vi "main.vi"() -> ()   [LabVIEW 2020]
uses:
  <vilib>/Platform/TimedLoop/XDataNode/timing_clust.ctl
  <vilib>/Platform/TimedLoop/XDataNode/nitl_modes.ctl
  <vilib>/Platform/TimedLoop/XDataNode/wakeup.ctl
  <vilib>/addons/control/pid/pid.llb/PID (DBL).vi
  <vilib>/imath/engines/lvmath2/RunTimeEngine/IndexReplace/NIMS M($,S)=V.vi
  <instcachedir>/0/NIMS M($,S)=V_85A28EB895514E96A13A10261726EE3A.lvgen/NIMS M($,S)=V_85A28EB895514E96A13A10261726EE3A_001.vi
  <vilib>/imathl/engines/lvmath/Functions/Error Handling/Create Error.vi
  <vilib>/imath/engines/lvmath2/RunTimeEngine/BuiltInFunctions/diag/NIMS_diag.vi
  <instcachedir>/0/NIMS_diag_5DC8FB40F025456A81838E2C880FD792.lvgen/NIMS_diag_5DC8FB40F025456A81838E2C880FD792_003.vi
  <vilib>/imath/engines/lvmath2/RunTimeEngine/NodeEndStatement/NIMS_NodeEndStatement_Output.vi
  <instcachedir>/0/NIMS_NodeEndStatement_Output_53EC0D466D134D7ABD903AC30B43404B.lvgen/NIMS_NodeEndStatement_Output_53EC0D466D134D7ABD903AC30B43404B_005.vi
  <instcachedir>/0/NIMS_NodeEndStatement_Output_53EC0D466D134D7ABD903AC30B43404B.lvgen/NIMS_NodeEndStatement_Output_53EC0D466D134D7ABD903AC30B43404B_010.vi
  <vilib>/imath/engines/lvmath2/RunTimeEngine/ErrorHandling/NIMS_Finalize Error.vi
  <vilib>/imath/engines/lvmath2/RunTimeEngine/IndexRead/NIMS V(S).vi
  <instcachedir>/0/NIMS V(S)_0488751826AF41519A22953C041130DC.lvgen/NIMS V(S)_0488751826AF41519A22953C041130DC_000.vi
  <vilib>/imath/engines/lvmath2/RunTimeEngine/ErrorHandling/NIMS_Create Error From Enums.vi
  <vilib>/imath/engines/lvmath2/RunTimeEngine/RangeToken/NIMS_Range_R2 - Integer.vi
  <instcachedir>/0/NIMS_Range_R2 - Integer_FFC1A4B1B9F04947ABCB56F009996D55.lvgen/NIMS_Range_R2 - Integer_FFC1A4B1B9F04947ABCB56F009996D55_000.vi
  <vilib>/imath/engines/lvmath2/RunTimeEngine/CommandStatement/MC_CommandStatement_break.vi
  <vilib>/imath/engines/lvmath2/RunTimeEngine/VariableToken/NIMS_VariableToken_CondDefinedDefinedByReplace.vi
  <instcachedir>/0/NIMS_VariableToken_CondDefinedDefinedByReplace_D162CFFC24174562A9FEA619A91E1A56.lvgen/NIMS_VariableToken_CondDefinedDefinedByReplace_D162CFFC24174562A9FEA619A91E1A56_000.vi
  <vilib>/imath/engines/lvmath2/RunTimeEngine/IndexReplace/NIMS V(S)=S.vi
  <instcachedir>/0/NIMS V(S)=S_36728E0438CF49488BD4AB9ABCA5ECA4.lvgen/NIMS V(S)=S_36728E0438CF49488BD4AB9ABCA5ECA4_001.vi
  <vilib>/imath/engines/lvmath2/RunTimeEngine/VariableToken/NIMS_VariableToken_CondDefined.vi
  <instcachedir>/0/NIMS_VariableToken_CondDefined_537E119D71C74F9D9452D6FF923F1E1F.lvgen/NIMS_VariableToken_CondDefined_537E119D71C74F9D9452D6FF923F1E1F_000.vi
  <vilib>/imath/engines/lvmath2/RunTimeEngine/IndexRead/NIMS V($).vi
  <instcachedir>/0/NIMS V($)_C593F32C7F6B43C7B1793952E292524F.lvgen/NIMS V($)_C593F32C7F6B43C7B1793952E292524F_000.vi
  <vilib>/imath/engines/lvmath2/RunTimeEngine/ArithmeticOperatorToken/NIMS_ArithmeticOperator_rightdiv(C,C).vi
  <instcachedir>/0/NIMS_ArithmeticOperator_rightdiv(C,C)_34A6183377BA4447889BB2F60308B12E.lvgen/NIMS_ArithmeticOperator_rightdiv(C,C)_34A6183377BA4447889BB2F60308B12E_000.vi
  <instcachedir>/0/NIMS_diag_5DC8FB40F025456A81838E2C880FD792.lvgen/NIMS_diag_5DC8FB40F025456A81838E2C880FD792_002.vi
  <vilib>/imath/engines/lvmath2/RunTimeEngine/ArithmeticOperatorToken/NIMS_ArithmeticOperator_minus.vi
  <instcachedir>/0/NIMS_ArithmeticOperator_minus_822089A08BE049DB927E6BEA78E100F1.lvgen/NIMS_ArithmeticOperator_minus_822089A08BE049DB927E6BEA78E100F1_009.vi
  <vilib>/imath/engines/lvmath2/RunTimeEngine/ArithmeticOperatorToken/NIMS_ArithmeticOperator_times.vi
  <instcachedir>/0/NIMS_ArithmeticOperator_times_E1747072C05B43E9AAEA71FEEAEB18C8.lvgen/NIMS_ArithmeticOperator_times_E1747072C05B43E9AAEA71FEEAEB18C8_002.vi
  <vilib>/imath/engines/lvmath2/RunTimeEngine/ArithmeticOperatorToken/NIMS_ArithmeticOperator_plus.vi
  <instcachedir>/0/NIMS_ArithmeticOperator_plus_54468E2FAC2848C4BF0D457641184E60.lvgen/NIMS_ArithmeticOperator_plus_54468E2FAC2848C4BF0D457641184E60_005.vi
  <instcachedir>/0/NIMS_ArithmeticOperator_minus_822089A08BE049DB927E6BEA78E100F1.lvgen/NIMS_ArithmeticOperator_minus_822089A08BE049DB927E6BEA78E100F1_004.vi
  <instcachedir>/0/NIMS_ArithmeticOperator_plus_54468E2FAC2848C4BF0D457641184E60.lvgen/NIMS_ArithmeticOperator_plus_54468E2FAC2848C4BF0D457641184E60_001.vi
  <instcachedir>/0/NIMS V($)_C593F32C7F6B43C7B1793952E292524F.lvgen/NIMS V($)_C593F32C7F6B43C7B1793952E292524F_001.vi
  <instcachedir>/0/NIMS_ArithmeticOperator_minus_822089A08BE049DB927E6BEA78E100F1.lvgen/NIMS_ArithmeticOperator_minus_822089A08BE049DB927E6BEA78E100F1_003.vi
  <instcachedir>/0/NIMS_ArithmeticOperator_plus_54468E2FAC2848C4BF0D457641184E60.lvgen/NIMS_ArithmeticOperator_plus_54468E2FAC2848C4BF0D457641184E60_004.vi
  <instcachedir>/0/NIMS V(S)=S_36728E0438CF49488BD4AB9ABCA5ECA4.lvgen/NIMS V(S)=S_36728E0438CF49488BD4AB9ABCA5ECA4_000.vi
  <instcachedir>/0/NIMS_ArithmeticOperator_times_E1747072C05B43E9AAEA71FEEAEB18C8.lvgen/NIMS_ArithmeticOperator_times_E1747072C05B43E9AAEA71FEEAEB18C8_000.vi
  <vilib>/imath/engines/lvmath2/RunTimeEngine/ArithmeticOperatorToken/NIMS_ArithmeticOperator_multmx(M,CV).vi
  <instcachedir>/0/NIMS_ArithmeticOperator_multmx(M,CV)_6A1ED936907E4DE39F29C31CF1EB9098.lvgen/NIMS_ArithmeticOperator_multmx(M,CV)_6A1ED936907E4DE39F29C31CF1EB9098_000.vi
  <vilib>/imath/engines/lvmath2/RunTimeEngine/ArithmeticOperatorToken/NIMS_ArithmeticOperator_multmx(M,CV)-internal.vi
  <instcachedir>/0/NIMS_ArithmeticOperator_multmx(M,CV)-internal_19A14CC5BE0A4D31BE1E94A2E998D8C3.lvgen/NIMS_ArithmeticOperator_multmx(M,CV)-internal_19A14CC5BE0A4D31BE1E94A2E998D8C3_001.vi
  <instcachedir>/0/NIMS_ArithmeticOperator_plus_54468E2FAC2848C4BF0D457641184E60.lvgen/NIMS_ArithmeticOperator_plus_54468E2FAC2848C4BF0D457641184E60_003.vi
  <instcachedir>/0/NIMS_ArithmeticOperator_plus_54468E2FAC2848C4BF0D457641184E60.lvgen/NIMS_ArithmeticOperator_plus_54468E2FAC2848C4BF0D457641184E60_010.vi
  <instcachedir>/0/NIMS_ArithmeticOperator_minus_822089A08BE049DB927E6BEA78E100F1.lvgen/NIMS_ArithmeticOperator_minus_822089A08BE049DB927E6BEA78E100F1_010.vi
  <vilib>/imath/engines/lvmath2/RunTimeEngine/ArithmeticOperatorToken/NIMS_ArithmeticOperator_multmx.vi
  <instcachedir>/0/NIMS_ArithmeticOperator_multmx_177F0753FB7A49B190E35F5DD0E80316.lvgen/NIMS_ArithmeticOperator_multmx_177F0753FB7A49B190E35F5DD0E80316_003.vi
  <instcachedir>/0/NIMS_ArithmeticOperator_multmx(M,CV)_6A1ED936907E4DE39F29C31CF1EB9098.lvgen/NIMS_ArithmeticOperator_multmx(M,CV)_6A1ED936907E4DE39F29C31CF1EB9098_003.vi
  <instcachedir>/0/NIMS_ArithmeticOperator_times_E1747072C05B43E9AAEA71FEEAEB18C8.lvgen/NIMS_ArithmeticOperator_times_E1747072C05B43E9AAEA71FEEAEB18C8_011.vi
  <instcachedir>/0/NIMS_ArithmeticOperator_plus_54468E2FAC2848C4BF0D457641184E60.lvgen/NIMS_ArithmeticOperator_plus_54468E2FAC2848C4BF0D457641184E60_002.vi
  <instcachedir>/0/NIMS_ArithmeticOperator_minus_822089A08BE049DB927E6BEA78E100F1.lvgen/NIMS_ArithmeticOperator_minus_822089A08BE049DB927E6BEA78E100F1_011.vi
  <vilib>/imath/engines/lvmath2/RunTimeEngine/ArithmeticOperatorToken/NIMS_ArithmeticOperator_rightdiv.vi
  <instcachedir>/0/NIMS_ArithmeticOperator_rightdiv_8260AC44E1124B869C886786403FE7FC.lvgen/NIMS_ArithmeticOperator_rightdiv_8260AC44E1124B869C886786403FE7FC_000.vi
  <instcachedir>/0/NIMS_ArithmeticOperator_multmx(M,CV)_6A1ED936907E4DE39F29C31CF1EB9098.lvgen/NIMS_ArithmeticOperator_multmx(M,CV)_6A1ED936907E4DE39F29C31CF1EB9098_001.vi
  <instcachedir>/0/NIMS_ArithmeticOperator_plus_54468E2FAC2848C4BF0D457641184E60.lvgen/NIMS_ArithmeticOperator_plus_54468E2FAC2848C4BF0D457641184E60_011.vi
  <instcachedir>/0/NIMS_ArithmeticOperator_minus_822089A08BE049DB927E6BEA78E100F1.lvgen/NIMS_ArithmeticOperator_minus_822089A08BE049DB927E6BEA78E100F1_008.vi
  <instcachedir>/0/NIMS_ArithmeticOperator_times_E1747072C05B43E9AAEA71FEEAEB18C8.lvgen/NIMS_ArithmeticOperator_times_E1747072C05B43E9AAEA71FEEAEB18C8_012.vi
  <instcachedir>/0/NIMS_ArithmeticOperator_rightdiv(C,C)_34A6183377BA4447889BB2F60308B12E.lvgen/NIMS_ArithmeticOperator_rightdiv(C,C)_34A6183377BA4447889BB2F60308B12E_001.vi
  <vilib>/imath/engines/lvmath2/RunTimeEngine/MatrixToken/NIMS_MatrixToken_SorCV_M.vi
  <instcachedir>/0/NIMS_MatrixToken_SorCV_M_84289C48EDA3463080C22A503926496B.lvgen/NIMS_MatrixToken_SorCV_M_84289C48EDA3463080C22A503926496B_000.vi
  <instcachedir>/0/NIMS_ArithmeticOperator_minus_822089A08BE049DB927E6BEA78E100F1.lvgen/NIMS_ArithmeticOperator_minus_822089A08BE049DB927E6BEA78E100F1_002.vi
  <instcachedir>/0/NIMS_MatrixToken_SorCV_M_84289C48EDA3463080C22A503926496B.lvgen/NIMS_MatrixToken_SorCV_M_84289C48EDA3463080C22A503926496B_001.vi
  <instcachedir>/0/NIMS_ArithmeticOperator_plus_54468E2FAC2848C4BF0D457641184E60.lvgen/NIMS_ArithmeticOperator_plus_54468E2FAC2848C4BF0D457641184E60_000.vi
  <vilib>/imath/engines/lvmath2/RunTimeEngine/IndexRead/NIMS V(R2).vi
  <instcachedir>/0/NIMS V(R2)_C76619605A0E4E9F8B2FA9389712AC47.lvgen/NIMS V(R2)_C76619605A0E4E9F8B2FA9389712AC47_000.vi
  <instcachedir>/0/NIMS V(R2)_C76619605A0E4E9F8B2FA9389712AC47.lvgen/NIMS V(R2)_C76619605A0E4E9F8B2FA9389712AC47_001.vi
  <vilib>/imath/engines/lvmath2/RunTimeEngine/BuiltInFunctions/reshapemx/NIMS_[GM]_reshapemx.vi
  <instcachedir>/0/NIMS_[GM]_reshapemx_98F4FEDA5D2741A4824CEDFB6097FB68.lvgen/NIMS_[GM]_reshapemx_98F4FEDA5D2741A4824CEDFB6097FB68_004.vi
  <vilib>/imath/engines/lvmath2/RunTimeEngine/IndexRead/NIMS M(S,$).vi
  <instcachedir>/0/NIMS M(S,$)_F24F360562DE41D8BE234322A2E15C65.lvgen/NIMS M(S,$)_F24F360562DE41D8BE234322A2E15C65_001.vi
  <vilib>/imath/engines/lvmath2/RunTimeEngine/ArithmeticOperatorToken/NIMS_ArithmeticOperator_multmx(RV,CV).vi
  <instcachedir>/0/NIMS_ArithmeticOperator_multmx(RV,CV)_B88EFA1B0B8541B182B3EADCEACED710.lvgen/NIMS_ArithmeticOperator_multmx(RV,CV)_B88EFA1B0B8541B182B3EADCEACED710_001.vi
  <instcachedir>/0/NIMS V(S)_0488751826AF41519A22953C041130DC.lvgen/NIMS V(S)_0488751826AF41519A22953C041130DC_003.vi
  <vilib>/imath/engines/lvmath2/RunTimeEngine/IndexReplace/NIMS V(S)=M.vi
  <instcachedir>/0/NIMS V(S)=M_4F924C5350174586BCA8F9B45EA0F965.lvgen/NIMS V(S)=M_4F924C5350174586BCA8F9B45EA0F965_001.vi
  <vilib>/imath/engines/lvmath2/RunTimeEngine/IndexRead/NIMS M(S).vi
  <instcachedir>/0/NIMS M(S)_B826C018497E4940AE96BD27B540B6FB.lvgen/NIMS M(S)_B826C018497E4940AE96BD27B540B6FB_004.vi
  <instcachedir>/0/NIMS_ArithmeticOperator_multmx(RV,CV)_B88EFA1B0B8541B182B3EADCEACED710.lvgen/NIMS_ArithmeticOperator_multmx(RV,CV)_B88EFA1B0B8541B182B3EADCEACED710_000.vi
  <vilib>/imath/engines/lvmath2/RunTimeEngine/ArithmeticOperatorToken/NIMS_ArithmeticOperator_rightdivmx(C,C).vi
  <instcachedir>/0/NIMS_ArithmeticOperator_rightdivmx(C,C)_00A7E666A69647418148ACDCFFBCE354.lvgen/NIMS_ArithmeticOperator_rightdivmx(C,C)_00A7E666A69647418148ACDCFFBCE354_000.vi
  <vilib>/imath/engines/lvmath2/RunTimeEngine/ArithmeticOperatorToken/NIMS_ArithmeticOperator_multmx(RV,CV)-internal.vi
  <instcachedir>/0/NIMS_ArithmeticOperator_multmx(RV,CV)-internal_E772CF64F86B43F3BAB2B4FC2EB32E29.lvgen/NIMS_ArithmeticOperator_multmx(RV,CV)-internal_E772CF64F86B43F3BAB2B4FC2EB32E29_002.vi
  <vilib>/imath/engines/lvmath2/RunTimeEngine/BuiltInFunctions/max/2 inputs/NIMS_max(CG,CG)-no size check.vi
  <instcachedir>/0/NIMS_max(CG,CG)-no size check_4775AE88A51C4793B48F105C5674D795.lvgen/NIMS_max(CG,CG)-no size check_4775AE88A51C4793B48F105C5674D795_000.vi
  <vilib>/imath/engines/lvmath2/RunTimeEngine/BuiltInFunctions/min/2 inputs/NIMS_min(CG,CG)-no size check.vi
  <instcachedir>/0/NIMS_min(CG,CG)-no size check_E9FF1D1EB4794D67BF6952418B074C1B.lvgen/NIMS_min(CG,CG)-no size check_E9FF1D1EB4794D67BF6952418B074C1B_000.vi
  <instcachedir>/0/NIMS V(S)_0488751826AF41519A22953C041130DC.lvgen/NIMS V(S)_0488751826AF41519A22953C041130DC_002.vi
  <instcachedir>/0/NIMS_max(CG,CG)-no size check_4775AE88A51C4793B48F105C5674D795.lvgen/NIMS_max(CG,CG)-no size check_4775AE88A51C4793B48F105C5674D795_001.vi
  <instcachedir>/0/NIMS_min(CG,CG)-no size check_E9FF1D1EB4794D67BF6952418B074C1B.lvgen/NIMS_min(CG,CG)-no size check_E9FF1D1EB4794D67BF6952418B074C1B_001.vi
  <instcachedir>/0/NIMS_diag_5DC8FB40F025456A81838E2C880FD792.lvgen/NIMS_diag_5DC8FB40F025456A81838E2C880FD792_004.vi
  <instcachedir>/0/NIMS_ArithmeticOperator_multmx_177F0753FB7A49B190E35F5DD0E80316.lvgen/NIMS_ArithmeticOperator_multmx_177F0753FB7A49B190E35F5DD0E80316_006.vi
  <instcachedir>/0/NIMS M(S)_B826C018497E4940AE96BD27B540B6FB.lvgen/NIMS M(S)_B826C018497E4940AE96BD27B540B6FB_000.vi
  <vilib>/imath/engines/lvmath2/RunTimeEngine/IndexReplace/NIMS M(S)=S.vi
  <instcachedir>/0/NIMS M(S)=S_033E230F5F1E47BAA81748F03F1A64B6.lvgen/NIMS M(S)=S_033E230F5F1E47BAA81748F03F1A64B6_001.vi
  <instcachedir>/0/NIMS M(S)=S_033E230F5F1E47BAA81748F03F1A64B6.lvgen/NIMS M(S)=S_033E230F5F1E47BAA81748F03F1A64B6_002.vi
  <instcachedir>/0/NIMS_ArithmeticOperator_times_E1747072C05B43E9AAEA71FEEAEB18C8.lvgen/NIMS_ArithmeticOperator_times_E1747072C05B43E9AAEA71FEEAEB18C8_003.vi
  <vilib>/imath/engines/lvmath2/RunTimeEngine/NodeEndStatement/NIMS_NodeEndStatement_Get Vector.vi
  <instcachedir>/0/NIMS_NodeEndStatement_Get Vector_F9EEA26507564AFBA1E30D500A99934B.lvgen/NIMS_NodeEndStatement_Get Vector_F9EEA26507564AFBA1E30D500A99934B_003.vi
  <instcachedir>/0/NIMS_NodeEndStatement_Get Vector_F9EEA26507564AFBA1E30D500A99934B.lvgen/NIMS_NodeEndStatement_Get Vector_F9EEA26507564AFBA1E30D500A99934B_001.vi
  <vilib>/imath/engines/lvmath2/RunTimeEngine/NodeEndStatement/NIMS_NodeEndStatement_Get Scalar.vi
  <instcachedir>/0/NIMS_NodeEndStatement_Get Scalar_52867EB063654D1B93D9FE1895BC48DF.lvgen/NIMS_NodeEndStatement_Get Scalar_52867EB063654D1B93D9FE1895BC48DF_000.vi
  <vilib>/imath/engines/lvmath/Functions/Error Handling/MergeErrorsWrapper.vi
  <instcachedir>/0/NIMS_NodeEndStatement_Output_53EC0D466D134D7ABD903AC30B43404B.lvgen/NIMS_NodeEndStatement_Output_53EC0D466D134D7ABD903AC30B43404B_000.vi
  <instcachedir>/0/NIMS_NodeEndStatement_Output_53EC0D466D134D7ABD903AC30B43404B.lvgen/NIMS_NodeEndStatement_Output_53EC0D466D134D7ABD903AC30B43404B_001.vi
  <instcachedir>/0/NIMS_NodeEndStatement_Output_53EC0D466D134D7ABD903AC30B43404B.lvgen/NIMS_NodeEndStatement_Output_53EC0D466D134D7ABD903AC30B43404B_009.vi
  <vilib>/Platform/TimedLoop/XDataNode/XDataNode.xnode
  <vilib>/Platform/TimedLoop/XDataNode/XDNodeRunTimeDep.lvlib
  <vilib>/addons/control/pid/NI_PID_pid.lvlib
panel:
  out "Gamma_L":dbl(graph)
  out "Load":dbl(graph)
  out "No error 3":bool
  out "No error 2":bool
  in  "Use\nPreset_Theta":bool=TRUE
  out "Theta_Boom_F_hat_next":T1(graph)
  out "Theta_Boom_Q_hat_next":T1(graph)
  out "Theta_Stick_Q_hat_next":T1(graph)
  out "Theta_Stick_F_hat_next":T1(graph)
  out "e2_e3":dbl[](array[numeric])
  out "e3":dbl[](array[numeric])
  out "e2":dbl[](array[numeric])
  out "F_Boom":cluster{dbl, dbl, dbl, dbl}(graph)
  out "Q_Swing":cluster{dbl, dbl, dbl, dbl}(graph)
  in  "保存路径":path=path "C:/Qmz/data1.bin"
  in  "Save Data":bool=TRUE
  in  "Stop\nTheta_Update":bool
  out "Q_Boom":cluster{dbl, dbl, dbl, dbl}(graph)
  out "F_Stick":cluster{dbl, dbl, dbl, dbl}(graph)
  out "Q_Stick":cluster{dbl, dbl, dbl, dbl}(graph)
  out "F_Swing":cluster{dbl, dbl, dbl, dbl}(graph)
  out "Esti_e2":T2(graph)={"FLda1[0]"=125.504748463915, "FLda1[1]"=53.955555282260676, "FLda1[2]"=-93.06627669799211}
  out "Esti_e1":T2(graph)={"FLda1[0]"=125.504748463915, "FLda1[1]"=53.955555282260676, "FLda1[2]"=-93.06627669799211}
  out "Swing":T3(graph)
  out "Stick":T3(graph)
  out "Boom":T3(graph)
  in  "sw_Y_Q":bool
  in  "w2":dbl[](array[numeric])=[1414.0, 4000.0, 3020.0]
  in  "w1":dbl[](array[numeric])=[0.26, 1.1, 0.07]
  out "Theta_Boom_Q_hat_next":dbl[](array[numeric])
  out "Theta_Boom_F_hat_next":dbl[](array[numeric])
  out "Theta_Swing_Q_hat_next":dbl[](array[numeric])
  out "Theta_Swing_F_hat_next":dbl[](array[numeric])
  out "Theta_Stick_Q_hat_next":dbl[](array[numeric])
  out "Theta_Stick_F_hat_next":dbl[](array[numeric])
  out "ARC_U":dbl[](array[numeric])
  in  "sw_d2hat":bool
  in  "sw_d1hat":bool
  in  "gamma_d2(E-8)":dbl[](array[numeric])=[6.5, 1.2, 3.5]
  in  "gamma_d1":dbl[](array[numeric])=[250.0, 6002.000000000004, 6000.1]
  in  "Theta_s2_init(E-8)":dbl[](array[numeric])=[2.0, 2.3, 2.5, 0.0, 100.0, 10.0, 0.0, -99.0, -200.0]
  in  "Theta_s1_init":dbl[](array[numeric])=[500.0, 66.0, 30.0, 53.0, 57.0, 31.0, -10.0, -73.0, 77.0]
  in  "sw_FLda1":bool=TRUE
  in  "sw_QLda1":bool=TRUE
  in  "STOP/Return to save position":bool=TRUE
  in  "Swing？(F)":bool=TRUE
  in  "Boom？(F)":bool
  in  "Stickj？(F)":bool=TRUE
  in  "K3(E-8)":dbl[](array[numeric])=[0.8, 1.0, 1.5] format="%#_8g"
  in  "K2":dbl[](array[numeric])=[650.0, 850.0, 790.0]
  in  "K1":dbl[](array[numeric])=[80.0, 80.0, 80.0]
  out "?":string="Now OpenLoop is running"
  out "?":string="Now OpenLoop is running"
  out "?":string="Now OpenLoop is running"
  in  "CloseLoop":T4 caption="ARC开关"
  out "Angle_Stick":dbl
  out "Angle_Boom":dbl
  out "Angle_Swing":dbl
  out "millisecond timer value":u32
  out "real time(s)":dbl
  out "minus":dbl format="%#_10g"
  out "No error":bool
  in  "PID gains":T5={"proportional gain (Kc)"=0.15, "integral time (Ti, min)"=0.003, "derivative time (Td, min)"=0.0005} caption="未越界" {"derivative time (Td, min)" format="%.6f"; "integral time (Ti, min)" format="%.6f"; "proportional gain (Kc)" step=0.01 format="%.6f"}
  out "?":bool
  in  "PID gains 2":T5={"proportional gain (Kc)"=0.16, "integral time (Ti, min)"=0.006, "derivative time (Td, min)"=0.0001} caption="未越界" {"derivative time (Td, min)" format="%.6f"; "integral time (Ti, min)" format="%.6f"; "proportional gain (Kc)" format="%.6f"}
  in  "PID gains 3":T5={"proportional gain (Kc)"=0.15, "integral time (Ti, min)"=0.003, "derivative time (Td, min)"=1e-05} caption="未越界" {"derivative time (Td, min)" step=0.001 format="%.6f"; "integral time (Ti, min)" step=0.001 format="%.6f"; "proportional gain (Kc)" step=0.01 format="%.6f"}
  out "?":bool
  out "?":bool
  in  "OpenLoop":T6={"Swing"=TRUE, "Boom"=TRUE, "Stick"=TRUE, "Swing_U"=-1.0, "Boom_U"=1.0, "Stick_U"=-1.0}
  in  "t-whole_Swing":i32=200
  in  "p_end Swing":dbl=-40.0
  in  "a_max Swing":dbl=-20.0
  in  "v_max Swing":dbl=-20.0
  in  "t-whole_Boom":i32=200
  in  "p_end Boom":dbl=-40.0
  in  "a_max Boom":dbl=-20.0
  in  "v_max Boom":dbl=-20.0
  in  "t-whole_Stick":i32=200
  in  "p_end_Stick":dbl=-20.0
  in  "a_max_Stick":dbl=-20.0
  in  "v_max_Stick":dbl=-20.0
  in  "pin1":dbl(slide)=-15.718390804597696 scale=-60.0..55.0
  in  "Stick":T7={"Open P2P Traj"=TRUE, "Open Sine Traj"=FALSE, "Open Ramp Traj"=FALSE, "Open DIY Traj"=FALSE}
  in  "Boom":T7={"Open P2P Traj"=TRUE, "Open Sine Traj"=FALSE, "Open Ramp Traj"=FALSE, "Open DIY Traj"=FALSE}
  in  "Swing":T7={"Open P2P Traj"=TRUE, "Open Sine Traj"=FALSE, "Open Ramp Traj"=FALSE, "Open DIY Traj"=FALSE}
  in  "pin2":dbl(slide)=69.49152542372882 scale=-20.0..90.0
  in  "pin3":dbl(slide)=-69.65868263473052 scale=-160.0..-53.0
  # "s1 上到下\nfv\nfc\nD_n\ns2 上到下\n1/beta\nD_Q1\nD_Q2"
  # "上到下\n*Ld \\ *Lda1 \\ *Lds2 \\ *Lda2"
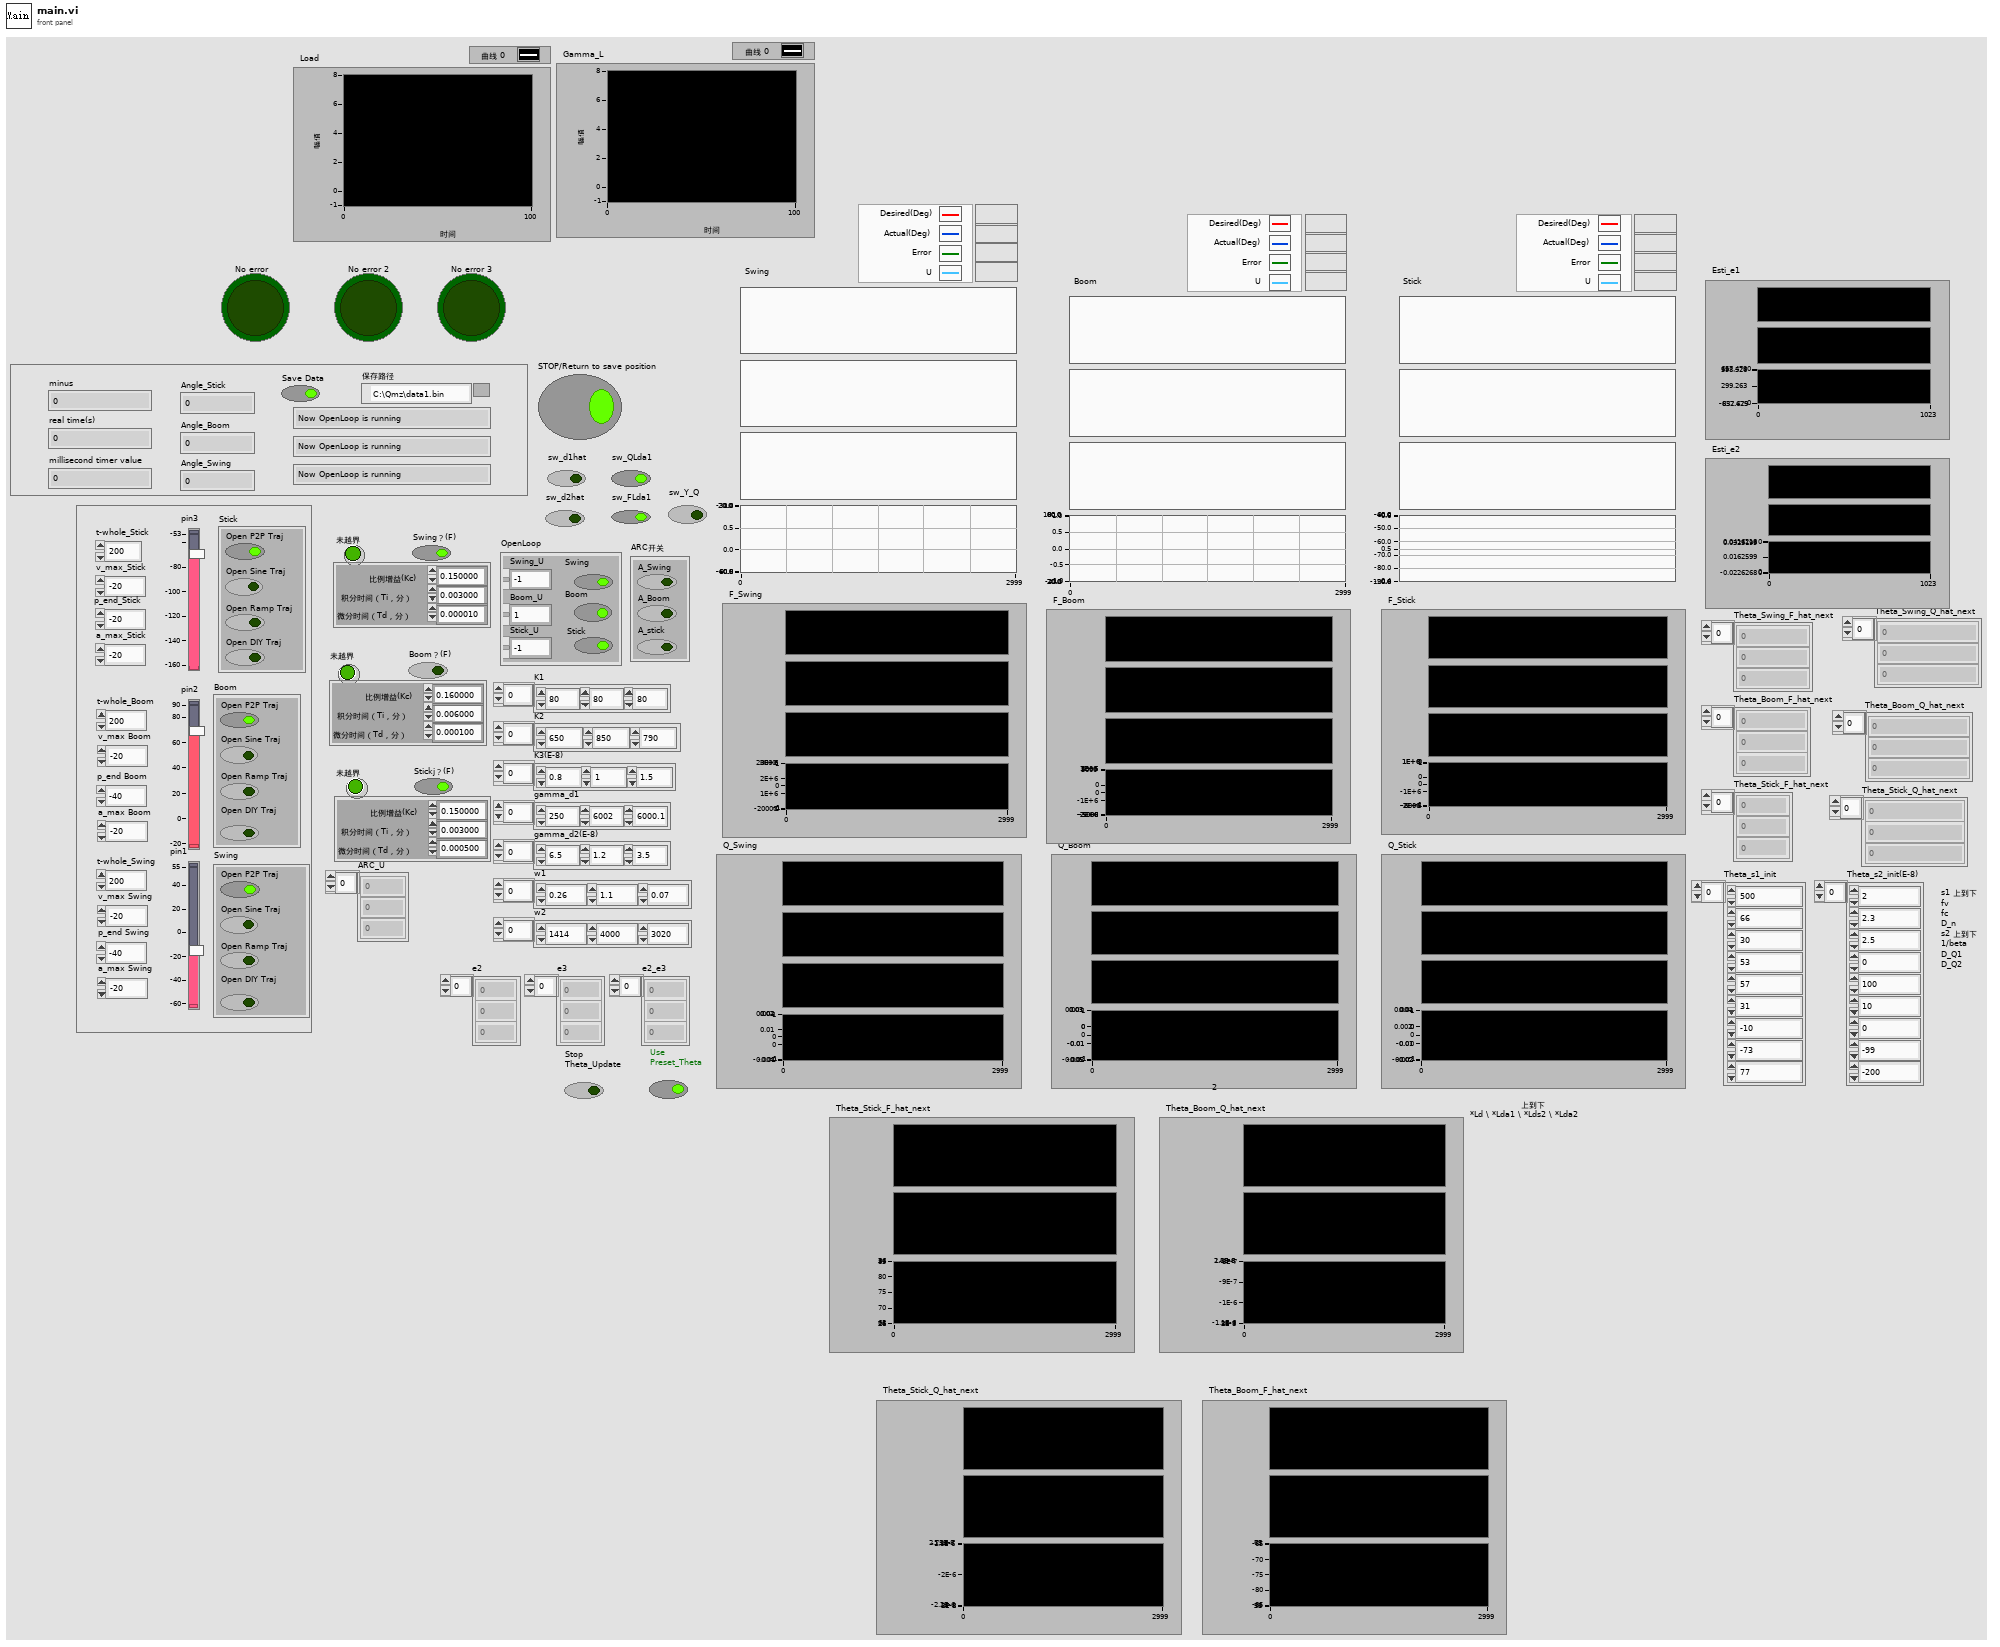
[diagram p1: front panel]
types:
  T1 = cluster{"Theta_Stick_F_hat_next[0]":dbl, "Theta_Stick_F_hat_next[1]":dbl, "Theta_Stick_F_hat_next[2]":dbl}
  T2 = cluster{"FLda1[0]":dbl, "FLda1[1]":dbl, "FLda1[2]":dbl}
  T3 = cluster{"Double":dbl, "Double":dbl, "Double":dbl, "Double":dbl}
  T4 = cluster{"A_Swing":bool, "A_Boom":bool, "A_stick\n":bool}
  T5 = cluster{"proportional gain (Kc)":dbl, "integral time (Ti, min)":dbl, "derivative time (Td, min)":dbl}
  T6 = cluster{"Swing":bool, "Boom":bool, "Stick":bool, "Swing_U":dbl, "Boom_U":dbl, "Stick_U":dbl}
  T7 = cluster{"Open P2P Traj":bool, "Open Sine Traj":bool, "Open Ramp Traj":bool, "Open DIY Traj":bool}
  T8 = typedef "XDNodeRunTimeDep.lvlib/timing_clust.ctl" = cluster{"Expected End [f-1]":u64, "Actual End [f-1]":u64, "Finished Late? [f-1]":bool, "Expected End [i-1]":u64, "Actual End [i-1]":u64, "Finished Late? [i-1]":bool, "Expected Start [i]":u64, "Actual Start [i]":u64, "Expected Start [f]":u64, "Actual Start [f]":u64, "Source Name":string, "Structure Name":string, "Period":i64, "Deadline":i64, "Offset":i64, "Start":i64, "Priority":i32, "Timeout":i32, "Mode":T9, "Wakeup Reason":T10, "Error":errorcluster, "Source Type":string, "Secondary Source Type":string, "Global End Time":u64, "Global Start Time":u64, "Frame Duration":u64, "Iteration Duration":u64, "Assigned CPU":i32, "I/O Scan Engine Mode":u32}
  T9 = typedef "XDNodeRunTimeDep.lvlib/nitl_modes.ctl" = enum32{"No Change", "Process missed periods, maintain original phase", "Discard missed periods, maintain original phase", "Process missed periods, ignore original phase", "Discard missed periods, ignore original phase"}
  T10 = typedef "XDNodeRunTimeDep.lvlib/wakeup.ctl" = enum32{"Normal", "Aborted", "Asynchronous wakeup", "Timing source error", "Timed loop error", "Timeout"}
  T11 = cluster{"Q_Stick[0]":cdb, "Q_Stick[1]":cdb, "Q_Stick[2]":cdb, "Q_Stick[3]":cdb}
  T12 = cluster{"Q_Boom[0]":cdb, "Q_Boom[1]":cdb, "Q_Boom[2]":cdb, "Q_Boom[3]":cdb}
  T13 = cluster{"Q_Swing[0]":cdb, "Q_Swing[1]":cdb, "Q_Swing[2]":cdb, "Q_Swing[3]":cdb}
  T14 = cluster{"F_Stick[0]":cdb, "F_Stick[1]":cdb, "F_Stick[2]":cdb, "F_Stick[3]":cdb}
  T15 = cluster{"F_Boom[0]":cdb, "F_Boom[1]":cdb, "F_Boom[2]":cdb, "F_Boom[3]":cdb}
  T16 = cluster{"F_Swing[0]":cdb, "F_Swing[1]":cdb, "F_Swing[2]":cdb, "F_Swing[3]":cdb}
  T17 = cluster{"Epsilon_1[0]":cdb, "Epsilon_1[1]":cdb, "Epsilon_1[2]":cdb}
  T18 = cluster{"Epsilon_2[0]":cdb, "Epsilon_2[1]":cdb, "Epsilon_2[2]":cdb}
  T19 = cluster{"Theta_Stick_Q_hat_next[0]":dbl, "Theta_Stick_Q_hat_next[1]":dbl, "Theta_Stick_Q_hat_next[2]":dbl}
  T20 = cluster{"Theta_Boom_Q_hat_next[0]":dbl, "Theta_Boom_Q_hat_next[1]":dbl, "Theta_Boom_Q_hat_next[2]":dbl}
  T21 = cluster{"Theta_Boom_F_hat_next[0]":dbl, "Theta_Boom_F_hat_next[1]":dbl, "Theta_Boom_F_hat_next[2]":dbl}
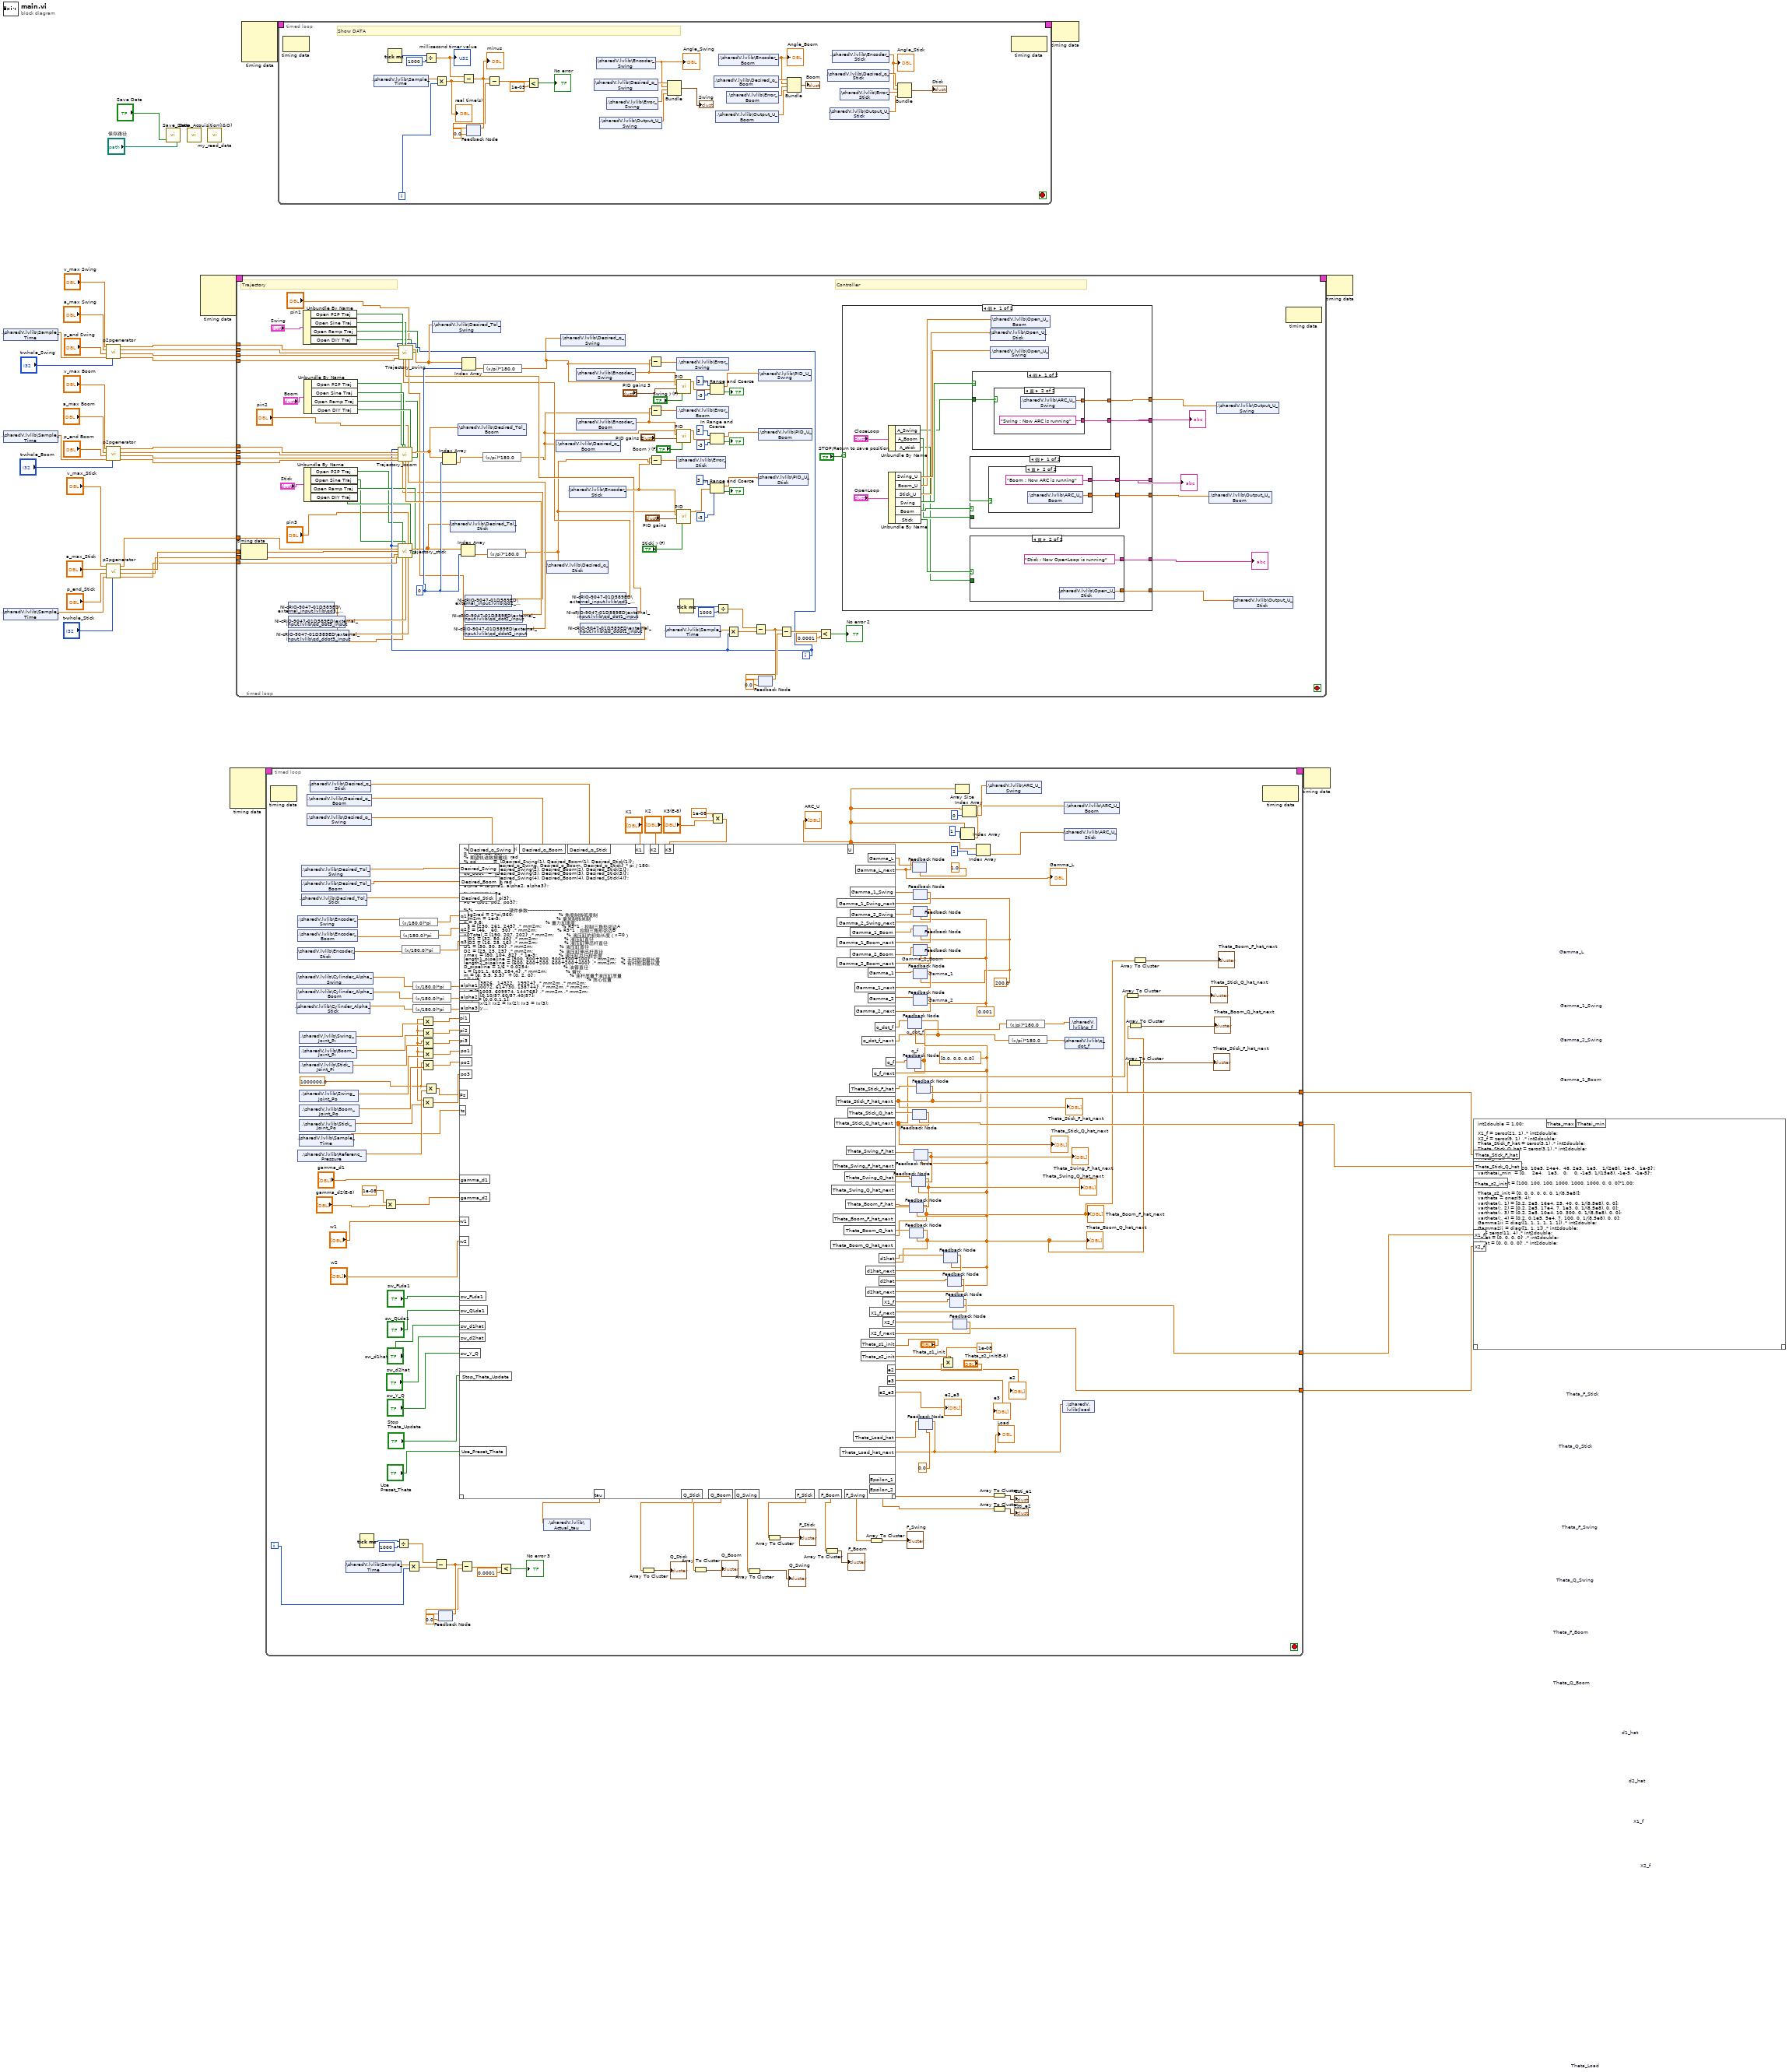
[diagram p0: block diagram]
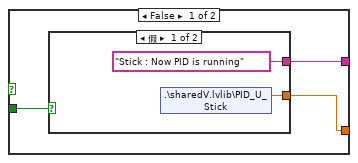
[diagram p2: hidden frame]
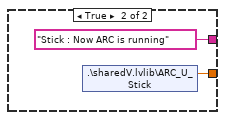
[diagram p3: hidden frame]
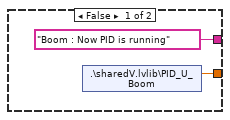
[diagram p4: hidden frame]
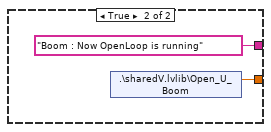
[diagram p5: hidden frame]
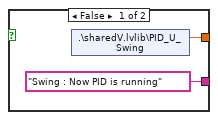
[diagram p6: hidden frame]
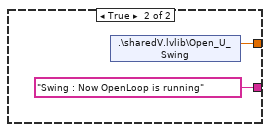
[diagram p7: hidden frame]
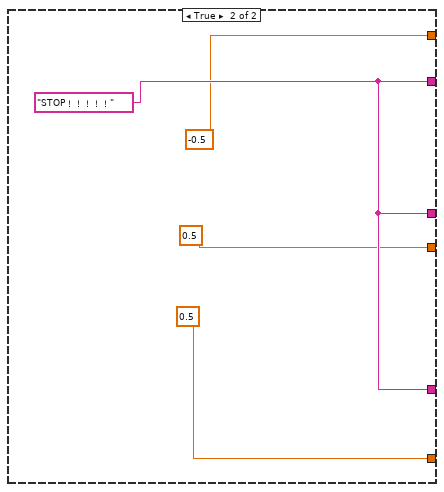
[diagram p8: hidden frame]
diagram:
  n1 = shared-variable ".\\sharedV.lvlib\\Sample_Time"() -> (w20:dbl)  [unwired: 1 in, 1 out]
  n2 = shared-variable ".\\sharedV.lvlib\\Sample_Time"() -> (w25:dbl)  [unwired: 1 in, 1 out]
  n3 = shared-variable ".\\sharedV.lvlib\\Sample_Time"() -> (w3:dbl)  [unwired: 1 in, 1 out]
  n4 = call "p2pgenerator.vi"("whole time for p2p"="t-whole_Swing", "ts"=w20, "p_end"="p_end Swing", "a_max"="a_max Swing", "v_max"="v_max Swing") -> ("jerk"=w12:dbl[], "a"=w13:dbl[], "v"=w14:dbl[], "s"=w15:dbl[])  [unwired: 3 in]
  n5 = call "p2pgenerator.vi"("whole time for p2p"="t-whole_Boom", "ts"=w25, "p_end"="p_end Boom", "a_max"="a_max Boom", "v_max"="v_max Boom") -> ("jerk"=w16:dbl[], "a"=w17:dbl[], "v"=w18:dbl[], "s"=w19:dbl[])  [unwired: 3 in]
  n6 = call "p2pgenerator.vi"("whole time for p2p"="t-whole_Stick", "ts"=w3, "p_end"="p_end_Stick", "a_max"="a_max_Stick", "v_max"="v_max_Stick") -> ("jerk"=w30:dbl[], "a"=w31:dbl[], "v"=w32:dbl[], "s"=w33:dbl[])  [unwired: 3 in]
  n7 = call "Save_Data.vi"("保存路径"="保存路径", "Save Data"="Save Data") -> ()  [unwired: 4 in]
  n8 = call "Data_Acquisition(I&O).vi"() -> ()  [unwired: 12 in]
  n9 = node-c288() -> (w39:T8)  [unwired: 4 in]
  n10 = call "my_read_data.vi"() -> ()  [unwired: 12 in]
  n11 = node-c288() -> (w9:T8)  [unwired: 4 in]
  n12 = timed-loop "定时循环" {
    timing: w39 -> [_]
    timing-out: [_] -> w38
    tunnel: w33 -> [w131]
    tunnel: w32 -> [w134]
    tunnel: w31 -> [w133]
    tunnel: w30 -> [w132]
    tunnel: w19 -> [w130]
    tunnel: w18 -> [w129]
    tunnel: w17 -> [w128]
    tunnel: w16 -> [w127]
    tunnel: w15 -> [w121]
    tunnel: w14 -> [w120]
    tunnel: w13 -> [w119]
    tunnel: w12 -> [w118]
    i -> [w59]
    stop <- _ stop-if-true
    w93 = 0
    # "Controller"
    # "Trajectory"
    n13 = node-c288() -> ()  [unwired: 1 in, 1 out]
    n14 = shared-variable "NI-cRIO-9047-01D589ED\\external_input.lvlib\\qd3_input"() -> (w48:dbl[])  [unwired: 1 in, 1 out]
    n15 = shared-variable "NI-cRIO-9047-01D589ED\\external_input.lvlib\\qd_dot3_input"() -> (w75:dbl[])  [unwired: 1 in, 1 out]
    n16 = shared-variable "NI-cRIO-9047-01D589ED\\external_input.lvlib\\qd_ddot3_input"() -> (w76:dbl[])  [unwired: 1 in, 1 out]
    n17 = Unbundle By Name ("按名称解除捆绑")("Swing") -> ("Open P2P Traj"=w123:bool, "Open Sine Traj"=w122:bool, "Open Ramp Traj"=w50:bool, "Open DIY Traj"=w49:bool)
    n18 = Unbundle By Name ("按名称解除捆绑")("Stick") -> ("Open P2P Traj"=w55:bool, "Open Sine Traj"=w56:bool, "Open Ramp Traj"=w57:bool, "Open DIY Traj"=w58:bool)
    n19 = Unbundle By Name ("按名称解除捆绑")("Boom") -> ("Open P2P Traj"=w52:bool, "Open Sine Traj"=w53:bool, "Open Ramp Traj"=w51:bool, "Open DIY Traj"=w54:bool)
    n20 = call "Trajectory_stick.vi"("i"=w59, "if p2p"=w55, "ifSin?"=w56, "Target_Angle"="pin3", "if_DIY"=w58, "q"=w131, "qd"=w134, "qdd"=w133, "if_Ramp"=w57, "qddd"=w132, "qd8_1"=w48, "qd8_dot_2"=w75, "qd8_ddot_2"=w76) -> ("qd1_tol"=w77:dbl[])  [unwired: 2 in]
    n21 = shared-variable ".\\sharedV.lvlib\\Desired_Tol_Stick"(w77) -> ()  [unwired: 1 in, 1 out]
    n22 = Index Array ("索引数组")(array=w77, index=w93) -> (element=w90:dbl)
    n23 = shared-variable "NI-cRIO-9047-01D589ED\\external_input.lvlib\\qd2_input"() -> (w47:dbl[])  [unwired: 1 in, 1 out]
    n24 = shared-variable "NI-cRIO-9047-01D589ED\\external_input.lvlib\\qd_dot2_input"() -> (w74:dbl[])  [unwired: 1 in, 1 out]
    n25 = shared-variable "NI-cRIO-9047-01D589ED\\external_input.lvlib\\qd_ddot2_input"() -> (w73:dbl[])  [unwired: 1 in, 1 out]
    n26 = call "Trajectory_boom.vi"("i"=w59, "if p2p"=w52, "ifSin?"=w53, "Target_Angle"="pin2", "if end8"=w54, "q"=w130, "qd"=w129, "qdd"=w128, "if  Ramp"=w51, "qddd"=w127, "qd8_1"=w47, "qd8_dot_2"=w74, "qd8_ddot_2"=w73) -> ("qd1_tol"=w97:dbl[])  [unwired: 2 in]
    n27 = Index Array ("索引数组")(array=w97, index=w93) -> (element=w96:dbl)
    n28 = shared-variable ".\\sharedV.lvlib\\Desired_Tol_Boom"(w97) -> ()  [unwired: 1 in, 1 out]
    n29 = expression code="(x/pi)*180.0" ("弧度转换至角度")(w96) -> (w42:dbl)
    n30 = expression code="(x/pi)*180.0" ("弧度转换至角度")(w90) -> (w41:dbl)
    n31 = shared-variable ".\\sharedV.lvlib\\Desired_q_Stick"(w41) -> ()  [unwired: 1 in, 1 out]
    n32 = shared-variable ".\\sharedV.lvlib\\Desired_q_Boom"(w42) -> ()  [unwired: 1 in, 1 out]
    n33 = shared-variable ".\\sharedV.lvlib\\Encoder_Stick"() -> (w85:dbl)  [unwired: 1 in, 1 out]
    n34 = shared-variable ".\\sharedV.lvlib\\Encoder_Swing"() -> (w83:dbl)  [unwired: 1 in, 1 out]
    n35 = shared-variable ".\\sharedV.lvlib\\Encoder_Boom"() -> (w84:dbl)  [unwired: 1 in, 1 out]
    n36 = shared-variable "NI-cRIO-9047-01D589ED\\external_input.lvlib\\qd1_input"() -> (w46:dbl[])  [unwired: 1 in, 1 out]
    n37 = shared-variable "NI-cRIO-9047-01D589ED\\external_input.lvlib\\qd_dot1_input"() -> (w72:dbl[])  [unwired: 1 in, 1 out]
    n38 = shared-variable "NI-cRIO-9047-01D589ED\\external_input.lvlib\\qd_ddot1_input"() -> (w71:dbl[])  [unwired: 1 in, 1 out]
    n39 = call "Trajectory_swing.vi"("i"=w59, "if p2p"=w123, "ifSin?"=w122, "Target_Angle"="pin1", "if end8"=w49, "q"=w121, "qd"=w120, "if Ramp"=w50, "qdd"=w119, "qddd"=w118, "qd8_1"=w46, "qd8_dot_2"=w72, "qd8_ddot_2"=w71) -> ("qd1_tol"=w94:dbl[])  [unwired: 2 in]
    n40 = shared-variable ".\\sharedV.lvlib\\Desired_Tol_Swing"(w94) -> ()  [unwired: 1 in, 1 out]
    n41 = Index Array ("索引数组")(array=w94, index=w93) -> (element=w92:dbl)
    n42 = expression code="(x/pi)*180.0" ("弧度转换至角度")(w92) -> (w40:dbl)
    n43 = shared-variable ".\\sharedV.lvlib\\Desired_q_Swing"(w40) -> ()  [unwired: 1 in, 1 out]
    n44 = Subtract ("减")(x=w83, y=w40) -> (x-y=w91:dbl)
    n45 = Subtract ("减")(x=w84, y=w42) -> (x-y=w95:dbl)
    n46 = Subtract ("减")(x=w85, y=w41) -> (x-y=w81:dbl)
    n47 = shared-variable ".\\sharedV.lvlib\\Sample_Time"() -> (w70:dbl)  [unwired: 1 in, 1 out]
    n48 = shared-variable ".\\sharedV.lvlib\\Error_Swing"(w91) -> ()  [unwired: 1 in, 1 out]
    n49 = call-poly <vilib>:"PID.vi"("reinitialize? (F)"="Swing？(F)", "PID gains"="PID gains 3", "process variable"=w83, "setpoint"=w40) -> ("output"=w117:dbl)  [unwired: 6 in, 1 out]
    n50 = shared-variable ".\\sharedV.lvlib\\Error_Boom"(w95) -> ()  [unwired: 1 in, 1 out]
    n51 = call-poly <vilib>:"PID.vi"("reinitialize? (F)"="Boom？(F)", "PID gains"="PID gains 2", "process variable"=w84, "setpoint"=w42) -> ("output"=w111:dbl)  [unwired: 6 in, 1 out]
    n52 = shared-variable ".\\sharedV.lvlib\\Error_Stick"(w81) -> ()  [unwired: 1 in, 1 out]
    n53 = call-poly <vilib>:"PID.vi"("reinitialize? (F)"="Stickj？(F)", "PID gains"="PID gains", "process variable"=w85, "setpoint"=w41) -> ("output"=w89:dbl)  [unwired: 6 in, 1 out]
    n54 = Tick Count (ms) ("时间计数器")() -> (millisecond timer value=w68:u32)
    n55 = In Range and Coerce ("判定范围并强制转换")(upper limit=3, x=w117, lower limit=-3) -> (coerced(x)=w101:dbl, In Range?=→"?":bool)
    n56 = In Range and Coerce ("判定范围并强制转换")(upper limit=3, x=w111, lower limit=-3) -> (coerced(x)=w102:dbl, In Range?=→"?":bool)
    n57 = In Range and Coerce ("判定范围并强制转换")(upper limit=3, x=w89, lower limit=-3) -> (coerced(x)=w103:dbl, In Range?=→"?":bool)
    n58 = Divide ("除")(x=w68, y=u32 1000) -> (x/y=w66:dbl)
    n59 = Multiply ("乘")(x=w70, y=w59) -> (x*y=w69:dbl)
    n60 = Subtract ("减")(x=w66, y=w69) -> (x-y=w62:dbl)
    n61 = shared-variable ".\\sharedV.lvlib\\PID_U_Swing"(w101) -> ()  [unwired: 1 in, 1 out]
    n62 = shared-variable ".\\sharedV.lvlib\\PID_U_Boom"(w102) -> ()  [unwired: 1 in, 1 out]
    n63 = shared-variable ".\\sharedV.lvlib\\PID_U_Stick"(w103) -> ()  [unwired: 1 in, 1 out]
    n64 = feedback #1 ("反馈节点")(0.0) -> (w61:dbl)
    n65 = feedback-in #1(w62) -> ()
    n66 = Subtract ("减")(x=w62, y=w61) -> (x-y=w65:dbl)
    n67 = Less? ("小于？")(x=w65, y=0.0001) -> (x < y?=→"No error 2":bool)
    n68 = case "条件结构" shown="假" "STOP/Return to save position" {
      tunnel: [w145 -0.5] -> w80
      tunnel: [w143 w182] -> w100
      tunnel: [w140 w182] -> w99
      tunnel: [w139 0.5] -> w79
      tunnel: [w138 w182] -> w98
      tunnel: [w137 0.5] -> w78
      frame False {
        n69 = Unbundle By Name ("按名称解除捆绑")("CloseLoop") -> ("A_Swing"=w144:bool, "A_Boom"=w141:bool, "A_stick"=w135:bool)
        n70 = Unbundle By Name ("按名称解除捆绑")("OpenLoop") -> ("Swing_U"=w150:dbl, "Boom_U"=w148:dbl, "Stick_U"=w147:dbl, "Swing"=w146:bool, "Boom"=w142:bool, "Stick"=w136:bool)
        n71 = case "条件结构" shown="假" w142 {
          tunnel: [w161 w169] -> w139
          tunnel: w141 -> [w163 _]
          tunnel: [w162 "Boom : Now OpenLoop is running"] -> w140
          frame False {
            n72 = case "条件结构" shown="真" w163 {
              tunnel: ["Boom : Now PID is running" "Boom : Now ARC is running"] -> w162
              tunnel: [w164 w166] -> w161
              frame False {
                n73 = shared-variable ".\\sharedV.lvlib\\PID_U_Boom"() -> (w164:dbl)  [unwired: 1 in, 1 out]
              }
              frame True {
                n74 = shared-variable ".\\sharedV.lvlib\\ARC_U_Boom"() -> (w166:dbl)  [unwired: 1 in, 1 out]
              }
            }
          }
          frame True {
            n75 = shared-variable ".\\sharedV.lvlib\\Open_U_Boom"() -> (w169:dbl)  [unwired: 1 in, 1 out]
          }
        }
        n76 = case "条件结构" shown="真" w136 {
          tunnel: [w152 w160] -> w137
          tunnel: w135 -> [w154 _]
          tunnel: [w153 "Stick : Now OpenLoop is running"] -> w138
          frame False {
            n77 = case "条件结构" shown="假" w154 {
              tunnel: ["Stick : Now PID is running" "Stick : Now ARC is running"] -> w153
              tunnel: [w155 w157] -> w152
              frame False {
                n78 = shared-variable ".\\sharedV.lvlib\\PID_U_Stick"() -> (w155:dbl)  [unwired: 1 in, 1 out]
              }
              frame True {
                n79 = shared-variable ".\\sharedV.lvlib\\ARC_U_Stick"() -> (w157:dbl)  [unwired: 1 in, 1 out]
              }
            }
          }
          frame True {
            n80 = shared-variable ".\\sharedV.lvlib\\Open_U_Stick"() -> (w160:dbl)  [unwired: 1 in, 1 out]
          }
        }
        n81 = case "条件结构" shown="假" w146 {
          tunnel: [w170 w178] -> w145
          tunnel: w144 -> [w172 _]
          tunnel: [w171 "Swing : Now OpenLoop is running"] -> w143
          frame False {
            n82 = case "条件结构" shown="真" w172 {
              tunnel: ["Swing : Now PID is running" "Swing : Now ARC is running"] -> w171
              tunnel: [w173 w175] -> w170
              frame False {
                n83 = shared-variable ".\\sharedV.lvlib\\PID_U_Swing"() -> (w173:dbl)  [unwired: 1 in, 1 out]
              }
              frame True {
                n84 = shared-variable ".\\sharedV.lvlib\\ARC_U_Swing"() -> (w175:dbl)  [unwired: 1 in, 1 out]
              }
            }
          }
          frame True {
            n85 = shared-variable ".\\sharedV.lvlib\\Open_U_Swing"() -> (w178:dbl)  [unwired: 1 in, 1 out]
          }
        }
        n86 = shared-variable ".\\sharedV.lvlib\\Open_U_Stick"(w147) -> ()  [unwired: 1 in, 1 out]
        n87 = shared-variable ".\\sharedV.lvlib\\Open_U_Swing"(w150) -> ()  [unwired: 1 in, 1 out]
        n88 = shared-variable ".\\sharedV.lvlib\\Open_U_Boom"(w148) -> ()  [unwired: 1 in, 1 out]
      }
      frame True {
        w182 = "STOP！！！！！"
      }
    }
    "?" <- w100
    "?" <- w99
    "?" <- w98
    n89 = shared-variable ".\\sharedV.lvlib\\Output_U_Boom"(w79) -> ()  [unwired: 1 in, 1 out]
    n90 = shared-variable ".\\sharedV.lvlib\\Output_U_Swing"(w80) -> ()  [unwired: 1 in, 1 out]
    n91 = shared-variable ".\\sharedV.lvlib\\Output_U_Stick"(w78) -> ()  [unwired: 1 in, 1 out]
    n92 = node-c288() -> ()  [unwired: 1 in, 1 out]
  }
  n93 = node-c288() -> (w11:T8)  [unwired: 4 in]
  n94 = timed-loop "定时循环" {
    timing: w11 -> [_]
    timing-out: [_] -> w10
    i -> [w200]
    stop <- _ stop-if-true
    # "Show DATA"
    n95 = node-c288() -> ()  [unwired: 1 in, 1 out]
    n96 = shared-variable ".\\sharedV.lvlib\\Sample_Time"() -> (w211:dbl)  [unwired: 1 in, 1 out]
    n97 = Tick Count (ms) ("时间计数器")() -> (millisecond timer value=w209:u32)
    n98 = Divide ("除")(x=w209, y=u32 1000) -> (x/y=w207:dbl)
    "millisecond timer value" <- w207
    n99 = Multiply ("乘")(x=w211, y=w200) -> (x*y=w210:dbl)
    "real time(s)" <- w210
    n100 = Subtract ("减")(x=w207, y=w210) -> (x-y=w203:dbl)
    "minus" <- w203
    n101 = feedback #2 ("反馈节点")(0.0) -> (w202:dbl)
    n102 = feedback-in #2(w203) -> ()
    n103 = Subtract ("减")(x=w203, y=w202) -> (x-y=w206:dbl)
    n104 = Less? ("小于？")(x=w206, y=1e-05) -> (x < y?=→"No error":bool)
    n105 = shared-variable ".\\sharedV.lvlib\\Desired_q_Swing"() -> (w199:dbl)  [unwired: 1 in, 1 out]
    n106 = shared-variable ".\\sharedV.lvlib\\Encoder_Swing"() -> (w191:dbl)  [unwired: 1 in, 1 out]
    "Angle_Swing" <- w191
    n107 = shared-variable ".\\sharedV.lvlib\\Output_U_Swing"() -> (w197:dbl)  [unwired: 1 in, 1 out]
    n108 = shared-variable ".\\sharedV.lvlib\\Error_Swing"() -> (w198:dbl)  [unwired: 1 in, 1 out]
    n109 = Bundle ("捆绑")("Double"=w199, "Double"=w191, "Double"=w198, "Double"=w197) -> (→"Swing":T3)  [unwired: 1 in]
    n110 = shared-variable ".\\sharedV.lvlib\\Desired_q_Boom"() -> (w195:dbl)  [unwired: 1 in, 1 out]
    n111 = shared-variable ".\\sharedV.lvlib\\Output_U_Boom"() -> (w192:dbl)  [unwired: 1 in, 1 out]
    n112 = shared-variable ".\\sharedV.lvlib\\Encoder_Boom"() -> (w194:dbl)  [unwired: 1 in, 1 out]
    "Angle_Boom" <- w194
    n113 = shared-variable ".\\sharedV.lvlib\\Error_Boom"() -> (w193:dbl)  [unwired: 1 in, 1 out]
    n114 = Bundle ("捆绑")("Double"=w195, "Double"=w194, "Double"=w193, "Double"=w192) -> (→"Boom":T3)  [unwired: 1 in]
    n115 = shared-variable ".\\sharedV.lvlib\\Desired_q_Stick"() -> (w188:dbl)  [unwired: 1 in, 1 out]
    n116 = shared-variable ".\\sharedV.lvlib\\Output_U_Stick"() -> (w190:dbl)  [unwired: 1 in, 1 out]
    n117 = shared-variable ".\\sharedV.lvlib\\Encoder_Stick"() -> (w187:dbl)  [unwired: 1 in, 1 out]
    "Angle_Stick" <- w187
    n118 = shared-variable ".\\sharedV.lvlib\\Error_Stick"() -> (w189:dbl)  [unwired: 1 in, 1 out]
    n119 = Bundle ("捆绑")("Double"=w188, "Double"=w187, "Double"=w189, "Double"=w190) -> (→"Stick":T3)  [unwired: 1 in]
    n120 = node-c288() -> ()  [unwired: 1 in, 1 out]
  }
  n121 = node-c288(w10) -> ()  [unwired: 1 out]
  n122 = node-c288(w38) -> ()  [unwired: 1 out]
  n123 = mathscript code="int2double = 1.00;\n\nX1_f = zeros(21, 1) .* int2double;\nX2_f = zeros(9, 1)  .* int2double;\nTheta_Stick_F_hat = zeros(3,1) .* int2double;\nTheta_Stick_Q_hat = zeros(3,1) .* int2double;\n\nTheta_max = 20;\nThetai_min  = -20;\nvarthetai_max = [20, 10e5, 24e4,  48, 2e3,  1e5,   1/(2e8),  1e-5,  1e-5]';\nvarthetai_min  = [0,    2e4,   1e3,   0,    0, -1e5, 1/(15e8), -1e-5,  -1e-5]';\n\nTheta_s1_init = [100, 100, 100, 1000, 1000, 1000, 0, 0, 0]*1.00;\n\nTheta_s2_init = [0, 0, 0, 0, 0, 0, 1/(8.5e8)];\nvartheta = ones(9, 4);\nvartheta(:, 1) = [0.2, 2e5, 16e4, 25, 40, 0, 1/(8.5e8), 0, 0];\nvartheta(:, 2) = [0.2, 2e5, 17e4, 7, 1e3, 0, 1/(8.5e8), 0, 0];\nvartheta(:, 3) = [0.2, 2e5, 10e4, 10, 300, 0, 1/(8.5e8), 0, 0];\nvartheta(:, 4) = [0.2, 0.1e5, 5e4, 7, 100, 0, 1/(8.5e8), 0, 0];\nGamma1ii = diag([1, 1, 1, 1, 1, 1]) .* int2double;\nGamma2ii = diag([1, 1, 1]) .* int2double;\nXf = zeros(11, 4) .* int2double;\ndihat = [0, 0, 0, 0]' .* int2double;\nzihat = [0, 0, 0, 0]' .* int2double;"() -> ("Theta_Stick_F_hat"=w5:dbl[], "X1_f"=w7:dbl[], "X2_f"=w6:dbl[], "Theta_Stick_Q_hat"=w4:dbl[])  [unwired: 1 in, 4 out]
  n124 = timed-loop "定时循环" {
    timing: w9 -> [_]
    timing-out: [_] -> w8
    tunnel: w7 -> [w301]
    tunnel: w6 -> [w300]
    tunnel: w5 -> [w298]
    tunnel: w4 -> [w296]
    i -> [w224]
    stop <- _ stop-if-true
    w251 = 0.001
    w250 = 200.0
    w266 = dbl[] [0.0, 0.0, 0.0]
    w341 = 1000000.0
    n125 = node-c288() -> ()  [unwired: 1 in, 1 out]
    n126 = shared-variable ".\\sharedV.lvlib\\Cylinder_Alpha_Swing"() -> (w362:dbl)  [unwired: 1 in, 1 out]
    n127 = shared-variable ".\\sharedV.lvlib\\Cylinder_Alpha_Boom"() -> (w359:dbl)  [unwired: 1 in, 1 out]
    n128 = shared-variable ".\\sharedV.lvlib\\Cylinder_Alpha_Stick"() -> (w358:dbl)  [unwired: 1 in, 1 out]
    n129 = shared-variable ".\\sharedV.lvlib\\Encoder_Swing"() -> (w340:dbl)  [unwired: 1 in, 1 out]
    n130 = shared-variable ".\\sharedV.lvlib\\Encoder_Boom"() -> (w339:dbl)  [unwired: 1 in, 1 out]
    n131 = shared-variable ".\\sharedV.lvlib\\Encoder_Stick"() -> (w338:dbl)  [unwired: 1 in, 1 out]
    n132 = shared-variable ".\\sharedV.lvlib\\Referenc_Pressure"() -> (w344:dbl)  [unwired: 1 in, 1 out]
    n133 = shared-variable ".\\sharedV.lvlib\\Swing_Joint_Pi"() -> (w356:dbl)  [unwired: 1 in, 1 out]
    n134 = shared-variable ".\\sharedV.lvlib\\Boom_Joint_Pi"() -> (w354:dbl)  [unwired: 1 in, 1 out]
    n135 = shared-variable ".\\sharedV.lvlib\\Stick_Joint_Pi"() -> (w353:dbl)  [unwired: 1 in, 1 out]
    n136 = shared-variable ".\\sharedV.lvlib\\Swing_Joint_Po"() -> (w352:dbl)  [unwired: 1 in, 1 out]
    n137 = shared-variable ".\\sharedV.lvlib\\Boom_Joint_Po"() -> (w351:dbl)  [unwired: 1 in, 1 out]
    n138 = shared-variable ".\\sharedV.lvlib\\Stick_Joint_Po"() -> (w336:dbl)  [unwired: 1 in, 1 out]
    n139 = shared-variable ".\\sharedV.lvlib\\Sample_Time"() -> (w337:dbl)  [unwired: 1 in, 1 out]
    n140 = shared-variable ".\\sharedV.lvlib\\Desired_Tol_Swing"() -> (w328:dbl[])  [unwired: 1 in, 1 out]
    n141 = shared-variable ".\\sharedV.lvlib\\Desired_Tol_Boom"() -> (w327:dbl[])  [unwired: 1 in, 1 out]
    n142 = shared-variable ".\\sharedV.lvlib\\Desired_Tol_Stick"() -> (w326:dbl[])  [unwired: 1 in, 1 out]
    n143 = shared-variable ".\\sharedV.lvlib\\Desired_q_Boom"() -> (w322:dbl)  [unwired: 1 in, 1 out]
    n144 = shared-variable ".\\sharedV.lvlib\\Desired_q_Swing"() -> (w321:dbl)  [unwired: 1 in, 1 out]
    n145 = shared-variable ".\\sharedV.lvlib\\Desired_q_Stick"() -> (w323:dbl)  [unwired: 1 in, 1 out]
    n146 = shared-variable ".\\sharedV.lvlib\\Sample_Time"() -> (w234:dbl)  [unwired: 1 in, 1 out]
    n147 = Tick Count (ms) ("时间计数器")() -> (millisecond timer value=w223:u32)
    n148 = Multiply ("乘")(x=1e-08, y="gamma_d2(E-8)") -> (x*y=w316:dbl[])
    n149 = Divide ("除")(x=w223, y=u32 1000) -> (x/y=w231:dbl)
    n150 = expression code="(x/180.0)*pi"(w340) -> (w363:dbl)
    n151 = expression code="(x/180.0)*pi"(w339) -> (w325:dbl)
    n152 = expression code="(x/180.0)*pi"(w338) -> (w324:dbl)
    n153 = Multiply ("乘")(x=w234, y=w224) -> (x*y=w233:dbl)
    n154 = expression code="(x/180.0)*pi"(w362) -> (w361:dbl)
    n155 = expression code="(x/180.0)*pi"(w359) -> (w360:dbl)
    n156 = expression code="(x/180.0)*pi"(w358) -> (w357:dbl)
    n157 = Multiply ("乘")(x=w341, y=w356) -> (x*y=w355:dbl)
    n158 = Multiply ("乘")(x=w341, y=w354) -> (x*y=w346:dbl)
    n159 = Multiply ("乘")(x=w341, y=w353) -> (x*y=w347:dbl)
    n160 = Multiply ("乘")(x=w341, y=w352) -> (x*y=w348:dbl)
    n161 = Multiply ("乘")(x=w341, y=w351) -> (x*y=w349:dbl)
    n162 = Multiply ("乘")(x=w341, y=w336) -> (x*y=w350:dbl)
    n163 = Multiply ("乘")(x=w341, y=w344) -> (x*y=w345:dbl)
    n164 = Subtract ("减")(x=w231, y=w233) -> (x-y=w227:dbl)
    n165 = feedback #3 ("反馈节点")(0.0) -> (w226:dbl)
    n166 = feedback-in #3(w227) -> ()
    n167 = Subtract ("减")(x=w227, y=w226) -> (x-y=w230:dbl)
    n168 = Less? ("小于？")(x=w230, y=0.0001) -> (x < y?=→"No error 3":bool)
    n169 = Multiply ("乘")(x=1e-08, y="K3(E-8)") -> (x*y=w313:dbl[])
    n170 = feedback #4 "q_f"(w266) -> (w268:dbl[])
    n171 = feedback #5 "q_dot_f"(w266) -> (w267:dbl[])
    n172 = feedback #6 "Theta_F_Boom"(w266) -> (w291:dbl[])
    n173 = feedback #7 "Theta_Q_Boom"(w266) -> (w290:dbl[])
    n174 = feedback #8 "Theta_Q_Swing"(w266) -> (w293:dbl[])
    n175 = feedback #9 "Theta_Q_Stick"(w296) -> (w297:dbl[])
    n176 = feedback #10 "Gamma_L"(1.0) -> (w219:cdb)
    n177 = feedback #11 "Gamma_1_Swing"(w250) -> (w263:dbl)
    n178 = feedback #12 "Gamma_2_Swing"(w251) -> (w261:dbl)
    n179 = feedback #13 "Gamma_1_Boom"(w250) -> (w259:dbl)
    n180 = feedback #14 "Gamma_2_Boom"(w251) -> (w257:dbl)
    n181 = feedback #15 "Gamma_1"(w250) -> (w255:dbl)
    n182 = feedback #16 "Gamma_2"(w251) -> (w253:dbl)
    n183 = feedback #17 "Theta_F_Swing"(w266) -> (w295:dbl[])
    n184 = feedback #18 "Theta_F_Stick"(w298) -> (w299:dbl[])
    n185 = feedback #19 "Theta_Load"(0.0) -> (w217:cdb)
    n186 = Multiply ("乘")(x=1e-08, y="Theta_s2_init(E-8)") -> (x*y=w306:dbl[])
    n187 = feedback #20 "d1_hat"(w266) -> (w312:dbl[])
    n188 = feedback #21 "d2_hat"(w266) -> (w310:dbl[])
    n189 = feedback #22 "X1_f"(w301) -> (w305:dbl[])
    n190 = feedback #23 "X2_f"(w300) -> (w304:dbl[])
    n191 = mathscript code="%%Author : Manzhi Qi\nq = [q1, q2, q3]';\n% 期望轨迹数据重组  rad\n% qd           =  [Desired_Swing(1), Desired_Boom(1), Desired_Stick(1)]';\nqd           =  [Desired_q_Swing, Desired_q_Boom, Desired_q_Stick]' * pi / 180;\nqd_dot     =  [Desired_Swing(2), Desired_Boom(2), Desired_Stick(2)]';\nqd_ddot   =  [Desired_Swing(3), Desired_Boom(3), Desired_Stick(3)]';\nqd_dddot =  [Desired_Swing(4), Desired_Boom(4), Desired_Stick(4)]';\n% 控制三角形夹角 rad\nalpha = [alpha1, alpha2, alpha3]'; \n\n% 液压缸压力 Pa\nPi = [pi1, pi2, pi3]';\nPo = [po1, po2, po3]';\n\n%% ----------------------硬件参数----------------------\ndeg2rad = 2*pi/360;                             % 角度制转弧度制\nmm2m = 1e-3;                                    % 毫米制转米制\ng = 9.8;                                        % 重力加速度\nAB = [230, 261, 245]' .* mm2m;             % R3*1：控制三角形邻边A\nBC = [46,   60,  50]' .* mm2m;             % R3*1：控制三角形邻边B\nx0Total = [190, 207, 202]' .* mm2m;        % 液压缸的初始长度（x=0）\n%D1 = [32, 50, 40]' .* mm2m;                 % 液压缸直径\n%D2 = [16, 25, 16]' .* mm2m;                 % 液压缸伸出杆直径\nD1 = [50, 50, 50]' .* mm2m;                 % 液压缸直径\nD2 = [25, 25, 25]' .* mm2m;                 % 液压缸伸出杆直径\nxmax = [80, 104, 82]' .* 1e-3;              % 液压缸总行程长度\nlength1_pipeline = [500, 500+300, 500+300+100]' .* mm2m;   % 无杆腔油管长度\nlength2_pipeline = [600, 600+200, 600+200+400]' .* mm2m;   % 有杆腔油管长度\nD_pipeline = 1/6 * 0.0254;                      % 油管直径\nL = [101.1, 605, 284.4]' .* mm2m;            % 臂长\nm = [6, 5.5, 3.3]'  + [0, 2, 0]';                      % 连杆质量+液压缸质量\nr = L/3;                                                                    % 质心位置\nIx = [13826,  14322,  19924]' .* mm2m .* mm2m;                        \nIy = [30072, 614730, 138744]' .* mm2m .* mm2m;                       \nIz = [21003, 609974, 144768]' .* mm2m .* mm2m;                       \n% q = [0,10/57,60/57,40/57];                                                \n% qd = [0,0,0.1,1];                                                      \nIx1 = Ix(1); Ix2 = Ix(2); Ix3 = Ix(3);\nIy1 = Iy(1); Iy2 = Iy(2); Iy3 = Iy(3);\nIz1 = Iz(1); Iz2 = Iz(2); Iz3 = Iz(3);\nm1 = m(1); m2 = m(2); m3 = m(3); \nr1 = r(1); r2 = r(2); r3 = r(3); \nL1 = L(1); L2 = L(2); L3 = L(3); \n\nfor ii = 1:3\n  xNowTotal(ii) = sqrt(AB(ii)^2 + BC(ii)^2 - 2*AB(ii)*BC(ii)*cos(alpha(ii)));           \t%控制三角形中关节角对应边长\nend\nxNowTotal = xNowTotal(:);\nJ_h = diag((AB .* BC .* sin(alpha)) ./ xNowTotal);\ninv_J_h = diag(xNowTotal./ (AB .* BC .* sin(alpha)));\n% 液压相关\nA_pipeline = 0.25*pi*D_pipeline^2;        \t        % 油管面积\nAi = 0.25*pi*D1.^2;                                 % 无杆腔面积\nAo = Ai - 0.25*pi*D2.^2;                      \t    % 有杆腔面积\nVh1 = A_pipeline .* length1_pipeline;               % 无杆腔油管油液体积\nVh2 = A_pipeline.*length2_pipeline + xmax.*Ao;      % 有杆腔油管油液体积\nxL = xNowTotal - x0Total;                           % 液压缸位移\nVi = Vh1 + Ai.*xL;                                  % 无杆腔油液总体积\nVo = Vh2 - Ao.*xL;                                  % 有杆腔油液总体积\nA_Q = Ai.^2./Vi + Ao.^2./Vo;\nB_Q = Ai ./ Vi;\nC_Q = Ao ./ Vo;\n\n% 二阶微分滤波求q_dot q_ddot.................\nq_dot_f = q_dot_f(:);\nq_f = q_f(:);\nq_dot = q_dot_f;\nwn = 80; % 原先是100，为了减少相位滞后，应当尽可能大\nepsilon = 0.707;\nq_ddot_f = wn^2*q - 2*epsilon*wn*q_dot_f - wn^2*q_f;\nq_dot_f_next = q_dot_f + q_ddot_f*ts;\nq_f_next = q_f + q_dot_f.*ts;\n\n%%\nq1d = q_dot(1);  q2d = q_dot(2);  q3d = q_dot(3); \nM =...\n[Ix2/2 + Ix3/2 + Iy2/2 + Iy3/2 + Iz1 - (Ix3*cos(2*q2 + 2*q3))/2 + (Iy3*cos(2*q2 + 2*q3))/2 + L1^2*m2 + L1^2*m3 + (L2^2*m3)/2 + (L3^2*m3)/2 + m1*r1^2 + (m2*r2^2)/2 - (Ix2*cos(2*q2))/2 + (Iy2*cos(2*q2))/2 + (L2^2*m3*cos(2*q2))/2 + (m2*r2^2*cos(2*q2))/2 + (L3^2*m3*cos(2*q2 + 2*q3))/2 + 2*L1*L3*m3*cos(q2 + q3) + 2*L1*L2*m3*cos(q2) + L2*L3*m3*cos(q3) + 2*L1*m2*r2*cos(q2) + L2*L3*m3*cos(2*q2 + q3),                                                            0,                                0;\n                                                                                                                                                                                                                                                                                                                                                                                                        0, m3*L2^2 + 2*m3*cos(q3)*L2*r3 + m2*r2^2 + m3*r3^2 + Iz2 + Iz3, m3*r3^2 + L2*m3*cos(q3)*r3 + Iz3;\n                                                                                                                                                                                                                                                                                                                                                                                                        0,                             m3*r3^2 + L2*m3*cos(q3)*r3 + Iz3,                    m3*r3^2 + Iz3];\n\nC =...\n[- q2d*((m3*sin(2*q2)*L2^2)/2 + m3*sin(2*q2 + q3)*L2*L3 + L1*m3*sin(q2)*L2 + (m3*sin(2*q2 + 2*q3)*L3^2)/2 + L1*m3*sin(q2 + q3)*L3 + (m2*sin(2*q2)*r2^2)/2 + L1*m2*sin(q2)*r2 - (Ix3*sin(2*q2 + 2*q3))/2 + (Iy3*sin(2*q2 + 2*q3))/2 - (Ix2*sin(2*q2))/2 + (Iy2*sin(2*q2))/2) - q3d*((Iy3*sin(2*q2 + 2*q3))/2 - (Ix3*sin(2*q2 + 2*q3))/2 + (L3^2*m3*sin(2*q2 + 2*q3))/2 + L1*L3*m3*sin(q2 + q3) + (L2*L3*m3*sin(q3))/2 + (L2*L3*m3*sin(2*q2 + q3))/2),  -q1d*((m3*sin(2*q2)*L2^2)/2 + m3*sin(2*q2 + q3)*L2*L3 + L1*m3*sin(q2)*L2 + (m3*sin(2*q2 + 2*q3)*L3^2)/2 + L1*m3*sin(q2 + q3)*L3 + (m2*sin(2*q2)*r2^2)/2 + L1*m2*sin(q2)*r2 - (Ix3*sin(2*q2 + 2*q3))/2 + (Iy3*sin(2*q2 + 2*q3))/2 - (Ix2*sin(2*q2))/2 + (Iy2*sin(2*q2))/2),  -q1d*((Iy3*sin(2*q2 + 2*q3))/2 - (Ix3*sin(2*q2 + 2*q3))/2 + (L3^2*m3*sin(2*q2 + 2*q3))/2 + L1*L3*m3*sin(q2 + q3) + (L2*L3*m3*sin(q3))/2 + (L2*L3*m3*sin(2*q2 + q3))/2);\n                                                                                                                                                                           q1d*((m3*sin(2*q2)*L2^2)/2 + m3*sin(2*q2 + q3)*L2*L3 + L1*m3*sin(q2)*L2 + (m3*sin(2*q2 + 2*q3)*L3^2)/2 + L1*m3*sin(q2 + q3)*L3 + (m2*sin(2*q2)*r2^2)/2 + L1*m2*sin(q2)*r2 - (Ix3*sin(2*q2 + 2*q3))/2 + (Iy3*sin(2*q2 + 2*q3))/2 - (Ix2*sin(2*q2))/2 + (Iy2*sin(2*q2))/2),                                                                                                                                                                                                                                                      -L2*m3*q3d*r3*sin(q3),                                                                                                                                           -L2*m3*r3*sin(q3)*(q2d + q3d);\n                                                                                                                                                                                                                                                                              q1d*((Iy3*sin(2*q2 + 2*q3))/2 - (Ix3*sin(2*q2 + 2*q3))/2 + (L3^2*m3*sin(2*q2 + 2*q3))/2 + L1*L3*m3*sin(q2 + q3) + (L2*L3*m3*sin(q3))/2 + (L2*L3*m3*sin(2*q2 + q3))/2),                                                                                                                                                                                                                                                       L2*m3*q2d*r3*sin(q3),                                                                                                                                                                       0;];\n\nG = [                                                    0;\n    g*(m2*r2*cos(q2) + m3*r3*cos(q2 + q3) + L2*m3*cos(q2));\n                                      g*m3*r3*cos(q2 + q3);] ;\n\n\nq1d_d = qd_dot(1);  q2d_d = qd_dot(2);  q3d_d = qd_dot(3); \nq1_d = qd(1);  q2_d = qd(2);  q3_d = qd(3); \nM_d =...\n[Ix2/2 + Ix3/2 + Iy2/2 + Iy3/2 + Iz1 - (Ix3*cos(2*q2_d + 2*q3_d))/2 + (Iy3*cos(2*q2_d + 2*q3_d))/2 + L1^2*m2 + L1^2*m3 + (L2^2*m3)/2 + (L3^2*m3)/2 + m1*r1^2 + (m2*r2^2)/2 - (Ix2*cos(2*q2_d))/2 + (Iy2*cos(2*q2_d))/2 + (L2^2*m3*cos(2*q2_d))/2 + (m2*r2^2*cos(2*q2_d))/2 + (L3^2*m3*cos(2*q2_d + 2*q3_d))/2 + 2*L1*L3*m3*cos(q2_d + q3_d) + 2*L1*L2*m3*cos(q2_d) + L2*L3*m3*cos(q3_d) + 2*L1*m2*r2*cos(q2_d) + L2*L3*m3*cos(2*q2_d + q3_d),                                                            0,                                0;\n                                                                                                                                                                                                                                                                                                                                                                                                        0, m3*L2^2 + 2*m3*cos(q3_d)*L2*r3 + m2*r2^2 + m3*r3^2 + Iz2 + Iz3, m3*r3^2 + L2*m3*cos(q3_d)*r3 + Iz3;\n                                                                                                                                                                                                                                                                                                                                                                                                        0,                             m3*r3^2 + L2*m3*cos(q3_d)*r3 + Iz3,                    m3*r3^2 + Iz3];\n\nC_d =...\n[- q2d_d*((m3*sin(2*q2_d)*L2^2)/2 + m3*sin(2*q2_d + q3_d)*L2*L3 + L1*m3*sin(q2_d)*L2 + (m3*sin(2*q2_d + 2*q3_d)*L3^2)/2 + L1*m3*sin(q2_d + q3_d)*L3 + (m2*sin(2*q2_d)*r2^2)/2 + L1*m2*sin(q2_d)*r2 - (Ix3*sin(2*q2_d + 2*q3_d))/2 + (Iy3*sin(2*q2_d + 2*q3_d))/2 - (Ix2*sin(2*q2_d))/2 + (Iy2*sin(2*q2_d))/2) - q3d_d*((Iy3*sin(2*q2_d + 2*q3_d))/2 - (Ix3*sin(2*q2_d + 2*q3_d))/2 + (L3^2*m3*sin(2*q2_d + 2*q3_d))/2 + L1*L3*m3*sin(q2_d + q3_d) + (L2*L3*m3*sin(q3_d))/2 + (L2*L3*m3*sin(2*q2_d + q3_d))/2),  -q1d_d*((m3*sin(2*q2_d)*L2^2)/2 + m3*sin(2*q2_d + q3_d)*L2*L3 + L1*m3*sin(q2_d)*L2 + (m3*sin(2*q2_d + 2*q3_d)*L3^2)/2 + L1*m3*sin(q2_d + q3_d)*L3 + (m2*sin(2*q2_d)*r2^2)/2 + L1*m2*sin(q2_d)*r2 - (Ix3*sin(2*q2_d + 2*q3_d))/2 + (Iy3*sin(2*q2_d + 2*q3_d))/2 - (Ix2*sin(2*q2_d))/2 + (Iy2*sin(2*q2_d))/2),  -q1d_d*((Iy3*sin(2*q2_d + 2*q3_d))/2 - (Ix3*sin(2*q2_d + 2*q3_d))/2 + (L3^2*m3*sin(2*q2_d + 2*q3_d))/2 + L1*L3*m3*sin(q2_d + q3_d) + (L2*L3*m3*sin(q3_d))/2 + (L2*L3*m3*sin(2*q2_d + q3_d))/2);\n                                                                                                                                                                           q1d_d*((m3*sin(2*q2_d)*L2^2)/2 + m3*sin(2*q2_d + q3_d)*L2*L3 + L1*m3*sin(q2_d)*L2 + (m3*sin(2*q2_d + 2*q3_d)*L3^2)/2 + L1*m3*sin(q2_d + q3_d)*L3 + (m2*sin(2*q2_d)*r2^2)/2 + L1*m2*sin(q2_d)*r2 - (Ix3*sin(2*q2_d + 2*q3_d))/2 + (Iy3*sin(2*q2_d + 2*q3_d))/2 - (Ix2*sin(2*q2_d))/2 + (Iy2*sin(2*q2_d))/2),                                                                                                                                                                                                                                                      -L2*m3*q3d_d*r3*sin(q3_d),                                                                                                                                           -L2*m3*r3*sin(q3_d)*(q2d_d + q3d_d);\n                                                                                                                                                                                                                                                                              q1d_d*((Iy3*sin(2*q2_d + 2*q3_d))/2 - (Ix3*sin(2*q2_d + 2*q3_d))/2 + (L3^2*m3*sin(2*q2_d + 2*q3_d))/2 + L1*L3*m3*sin(q2_d + q3_d) + (L2*L3*m3*sin(q3_d))/2 + (L2*L3*m3*sin(2*q2_d + q3_d))/2),                                                                                                                                                                                                                                                       L2*m3*q2d_d*r3*sin(q3_d),                                                                                                                                                                       0;];\n\nG_d = [                                                    0;\n    g*(m2*r2*cos(q2_d) + m3*r3*cos(q2_d + q3_d) + L2*m3*cos(q2_d));\n                                      g*m3*r3*cos(q2_d + q3_d);] ;\n\nM_load = [\n    (L2^2*cos(2*q2))/2 + (L3^2*cos(2*q2 + 2*q3))/2 + L1^2 + L2^2/2 + L3^2/2 + 2*L1*L3*cos(q2 + q3) + 2*L1*L2*cos(q2) + L2*L3*cos(q3) + L2*L3*cos(2*q2 + q3), 0, 0;\n    0, L2^2 + 2*cos(q3)*L2*L3 + L3^2, L3^2 + L2*cos(q3)*L3;\n    0, L3^2 + L2*cos(q3)*L3, L3^2\n];\n\nC_load= [\n - (L2^2*q2d*sin(2*q2))/2 - (L3^2*q2d*sin(2*q2 + 2*q3))/2 - (L3^2*q3d*sin(2*q2 + 2*q3))/2 - L1*L3*q2d*sin(q2 + q3) - L1*L3*q3d*sin(q2 + q3) - L1*L2*q2d*sin(q2) - (L2*L3*q3d*sin(q3))/2 - L2*L3*q2d*sin(2*q2 + q3) - (L2*L3*q3d*sin(2*q2 + q3))/2, -(q1d*(sin(2*q2)*L2^2 + 2*sin(2*q2 + q3)*L2*L3 + 2*L1*sin(q2)*L2 + sin(2*q2 + 2*q3)*L3^2 + 2*L1*sin(q2 + q3)*L3))/2, -(L3*q1d*(L3*sin(2*q2 + 2*q3) + 2*L1*sin(q2 + q3) + L2*sin(q3) + L2*sin(2*q2 + q3)))/2;\n   (q1d*(sin(2*q2)*L2^2 + 2*sin(2*q2 + q3)*L2*L3 + 2*L1*sin(q2)*L2 + sin(2*q2 + 2*q3)*L3^2 + 2*L1*sin(q2 + q3)*L3))/2, -L2*L3*q3d*sin(q3), -L2*L3*sin(q3)*(q2d + q3d);\n   (L3*q1d*(L3*sin(2*q2 + 2*q3) + 2*L1*sin(q2 + q3) + L2*sin(q3) + L2*sin(2*q2 + q3)))/2, L2*L3*q2d*sin(q3), 0\n];\n\nG_load = [                               0;\n                L3*g*cos(q2 + q3) + L2*g*cos(q2);\n                       L3*g*cos(q2 + q3); ];\n\n\n%% Update\nTheta_s1_init = Theta_s1_init(:);\nTheta_s2_init = Theta_s2_init(:);\n%% 预处理\ntheta_hat1 = zeros(3,1);\ntheta_hat2 = zeros(3,1);\ntheta_hat3 = zeros(3,1);\ntheta_hat4 = zeros(3,1);\ntheta_hat5 = zeros(3,1);\ntheta_hat6 = zeros(3,1);\n\ntheta_hat1 (1) = Theta_Swing_F_hat (1); % fv\ntheta_hat2 (1) = Theta_Swing_F_hat (2); % fc\ntheta_hat3 (1) = Theta_Swing_F_hat (3); % D_Fn\ntheta_hat4 (1) = Theta_Swing_Q_hat (1); % 1/beta_e\ntheta_hat5 (1) = Theta_Swing_Q_hat (2); % D_Qin\ntheta_hat6 (1) = Theta_Swing_Q_hat (3); % D_Qon\n\ntheta_hat1 (2) = Theta_Boom_F_hat (1);\ntheta_hat2 (2) = Theta_Boom_F_hat (2);\ntheta_hat3 (2) = Theta_Boom_F_hat (3);\ntheta_hat4 (2) = Theta_Boom_Q_hat (1);\ntheta_hat5 (2) = Theta_Boom_Q_hat (2);\ntheta_hat6 (2) = Theta_Boom_Q_hat (3);\n\ntheta_hat1 (3) = Theta_Stick_F_hat (1);\ntheta_hat2 (3) = Theta_Stick_F_hat (2);\ntheta_hat3 (3) = Theta_Stick_F_hat (3);\ntheta_hat4 (3) = Theta_Stick_Q_hat (1);\ntheta_hat5 (3) = Theta_Stick_Q_hat (2);\ntheta_hat6 (3) = Theta_Stick_Q_hat (3);\n\n\n%% step1\nK1 = K1(:);\nK2 = K2(:);\nK3 = K3(:);\ne1 = q - qd;\ne1_dot = q_dot - qd_dot;\nqeq_dot = qd_dot - K1.*e1;\nqeq_ddot = qd_ddot - K1.*e1_dot;\ne2 = q_dot - qeq_dot;\nS_qdot = 2/pi*atan(900*q_dot);   \nSd_qdot = 2/pi*atan(900*qd_dot);   \n\nFLda1 = inv_J_h * (M_d * qeq_dot + C_d * qd_dot + G_d + theta_hat1 .* qd_dot + theta_hat2 .* Sd_qdot - theta_hat3);\nFLds1 = - inv_J_h * K2 .* e2;\nFLda2 = - inv_J_h * d1hat(:);\nFLds2 = 0;\n\nFLd = FLda1* sw_FLda1 + FLda2  + FLds1 + FLds2;\nFL = Pi.*Ai - Po.*Ao; \ne3 = FL - FLd;\n%% step2\nFLdc_dot = zeros(3,1);\n\n% QLda1 = J_h*A_Q*q_dot - B_Q*theta_hat4 - C_Q*theta_hat5 + FLdc_dot*theta_hat6 + Upsilon_Q;\nw1 = w1( : ) ;\nw2 = w2 ( : ); \nomega = w1 ./ w2 ;\n\nQLda1 = J_h*diag(A_Q) * qd_dot + diag(FLdc_dot) * theta_hat4 - diag(B_Q) * theta_hat5 - diag(C_Q) * theta_hat6 ;\nQLda2 = -d2hat( : );\nQLds1 = -K3 .* e3;     \nY_Q = -J_h * omega .* e2 * sw_Y_Q;                                    \nQLd = QLda1 * sw_QLda1 + QLda2  +  QLds1  + Y_Q; \ne2_e3 = e2./e3;\n\n\n%% ----------------------Filtering----------------------\ntau_f = 0.006 ;                                    % Low-pass time constant (s)\n% ---------- 1) First-order regressors ----------\ntemp_A  = [q_dot;                                  % 3×1  Joint velocities\n           S_qdot;                                 % 3×1  Saturated velocities\n           -ones(3,1);                             % 3×1  Constant term\n           B_Q;                                    % 3×1  Flow-pressure coeffs\n           C_Q;                                    % 3×1  Flow-leakage coeffs\n           J_h*FL + C'*q_dot - G;                  % 3×1  Arm-side dynamics\n           C_load'*q_dot - G_load];                % 3×1  Load-side dynamics\n% ---------- 2) Output signals ----------\ntemp_B = [FL;                                  % 3×1  Load pressures\n          M*q_dot;                             % 3×1  Arm momentum\n          M_load*q_dot];                       % 3×1  Load momentum\n% Normal Filiter\nX1_f_next = (temp_A - X1_f( : )) / tau_f * ts + X1_f( : );\n% first-order Filiter\nX2_f_next = (temp_B - X2_f( : )) / tau_f * ts + X2_f( : ) ;\ntemp_B_dot  = (temp_B - X2_f( : )) / tau_f ;\n\nfilter_FL_dot     =  temp_B_dot(1 : 3);\nfilter_P_dot      =  temp_B_dot(4 : 6);\nfilter_P_Load_dot =  temp_B_dot(7 : 9);\n\n% ---------- 3) Dynamics regressor ----------\nA_f     = X1_f_next(16:18);                     % 3×1  Arm-side dynamics term\nB_Q_f   = X1_f_next(10:12);                     % 3×1  Filtered B_Q\nC_Q_f   = X1_f_next(13:15);                     % 3×1  Filtered C_Q\n\nu1f_phi = filter_P_dot - A_f;\nu2f_phi = QLd - J_h * diag(A_Q) * q_dot; \n\nphi1f = reshape( X1_f_next ( 1 : 9 ) , 3 , 3 ) ;   % Arrange by column q_dot / S_qdot / - ones(3,1)\ntemp =  [ -filter_FL_dot ; B_Q_f ; C_Q_f ];\nphi2f = reshape( temp  , 3 , 3 ) ; % Arrange by column -FL_dot / B_Q / C_Q\n\n% ----------------------Load_part----------------------\nF_V = [50,50,50]';\nF_S = [100, 100, 100]';\nT_ff = F_V.* X1_f_next(1:3) + F_S .* X1_f_next(4:6);\nu_load_f_phi = filter_P_dot - A_f + T_ff;\nu_load_f_phi = u_load_f_phi*(-1);\nphi_load_f = X1_f_next(19:21) - filter_P_Load_dot;\n\n%%  ----------------------Theta_Updata----------------------\nF_Phi_Swing = phi1f ( 1 , : )';\nQ_Phi_Swing = phi2f ( 1 , : )';\nF_Phi_Boom= phi1f ( 2 , : )';\nQ_Phi_Boom = phi2f ( 2 , : )';\nF_Phi_Stick = phi1f ( 3 , : )';\nQ_Phi_Stick = phi2f ( 3 , : )';\n%Theta_Stick_hat = zeros(3,1);\nTheta_Swing_F_hat = Theta_Swing_F_hat( : );\nTheta_Swing_Q_hat = Theta_Swing_Q_hat( : );\nTheta_Boom_F_hat = Theta_Boom_F_hat( : );\nTheta_Boom_Q_hat = Theta_Boom_Q_hat( : );\nTheta_Stick_F_hat = Theta_Stick_F_hat( : );\nTheta_Stick_Q_hat = Theta_Stick_Q_hat( : );\nTheta_Load_hat = 0;\nv1 = 0.1;\nv2 = 0.1;\nv_L = 0.1;\n% Calculate estimation errors Epsilon\nEpsilon_1 = zeros(3, 1);\nEpsilon_2 = zeros(3, 1);\n\nEpsilon_1(1) = -F_Phi_Swing' * Theta_Swing_F_hat - u1f_phi(1);   % Swing\nEpsilon_1(2) = -F_Phi_Boom' * Theta_Boom_F_hat - u1f_phi(2);     % Boom\nEpsilon_1(3) = -F_Phi_Stick' * Theta_Stick_F_hat - u1f_phi(3);   % Stick\n\nEpsilon_2(1) = -Q_Phi_Swing' * Theta_Swing_Q_hat - u2f_phi(1);   % Swing\nEpsilon_2(2) = -Q_Phi_Boom' * Theta_Boom_Q_hat - u2f_phi(2);     % Boom\nEpsilon_2(3) = -Q_Phi_Stick' * Theta_Stick_Q_hat - u2f_phi(3);   % Stick\n\nEpsilon_load = -phi_load_f * Theta_Load_hat - u_load_f_phi;      % 3*1\n\n% Calculate xi\nxi_1 = zeros(3, 1);\nxi_2 = zeros(3, 1);\nxi_1(1) = 1 / (1 + v1 * F_Phi_Swing' * Gamma_1_Swing * F_Phi_Swing);  % Swing\nxi_1(2) = 1 / (1 + v1 * F_Phi_Boom' * Gamma_1_Boom * F_Phi_Boom);     % Boom\nxi_1(3) = 1 / (1 + v1 * F_Phi_Stick' * Gamma_1 * F_Phi_Stick);        % Stick\n\nxi_2(1) = 1 / (1 + v2 * Q_Phi_Swing' * Gamma_2_Swing * Q_Phi_Swing);  % Swing\nxi_2(2) = 1 / (1 + v2 * Q_Phi_Boom' * Gamma_2_Boom * Q_Phi_Boom);     % Boom\nxi_2(3) = 1 / (1 + v2 * Q_Phi_Stick' * Gamma_2 * Q_Phi_Stick);        % Stick\n\nxi_L = 1 / (1 + v_L * phi_load_f' * Gamma_L * phi_load_f);           % Load\n\n% Since tau vectors might have different dimensions, store them separately\ntau_1_Swing = xi_1(1) * F_Phi_Swing * Epsilon_1(1);  % Swing\ntau_1_Boom = xi_1(2) * F_Phi_Boom * Epsilon_1(2);    % Boom\ntau_1_Stick = xi_1(3) * F_Phi_Stick * Epsilon_1(3);  % Stick\n\ntau_2_Swing = xi_2(1) * Q_Phi_Swing * Epsilon_2(1);  % Swing\ntau_2_Boom = xi_2(2) * Q_Phi_Boom * Epsilon_2(2);    % Boom\ntau_2_Stick = xi_2(3) * Q_Phi_Stick * Epsilon_2(3);  % Stick\n\ntau_Load = xi_L * phi_load_f' * Epsilon_load;  % Load\n\n% Calculate derivatives of Theta_hat\nTheta_Swing_F_hat_dot = Gamma_1_Swing * tau_1_Swing;  % Swing\nTheta_Boom_F_hat_dot = Gamma_1_Boom * tau_1_Boom;     % Boom\nTheta_Stick_F_hat_dot = Gamma_1 * tau_1_Stick;        % Stick\n\nTheta_Swing_Q_hat_dot = Gamma_2_Swing * tau_2_Swing;  % Swing\nTheta_Boom_Q_hat_dot = Gamma_2_Boom * tau_2_Boom;     % Boom\nTheta_Stick_Q_hat_dot = Gamma_2 * tau_2_Stick;        % Stick\n\nTheta_Load_hat_dot = Gamma_L * tau_Load;        % LOad\n%Theta_Load_hat_dot = 1* tau_Load;        % LOad\n\n% Calculate Theta_hat for next time step\nTheta_Swing_F_hat_next = Theta_Swing_F_hat_dot * ts + Theta_Swing_F_hat;  % Swing\nTheta_Boom_F_hat_next = Theta_Boom_F_hat_dot * ts + Theta_Boom_F_hat;     % Boom\nTheta_Stick_F_hat_next = Theta_Stick_F_hat_dot * ts + Theta_Stick_F_hat;  % Stick\n\nTheta_Swing_Q_hat_next = Theta_Swing_Q_hat_dot * ts + Theta_Swing_Q_hat;  % Swing\nTheta_Boom_Q_hat_next = Theta_Boom_Q_hat_dot * ts + Theta_Boom_Q_hat;     % Boom\nTheta_Stick_Q_hat_next = Theta_Stick_Q_hat_dot * ts + Theta_Stick_Q_hat;  % Stick\n\nTheta_Load_hat_next  = Theta_Load_hat_dot * ts + Theta_Load_hat;\n\n% Parameter limits\nTheta_Swing_Max = [100, 500, 200, 1/(2e8), 1e-5, 1e-5];  % fv fc D_Fn D_Qin D_Qon 1/beta\nTheta_Swing_Min = [10,   20, -200, 1/(1.25e9), -1e-5, -1e-5];\nTheta_Boom_Max = [100, 500, 200, 1/(2e8), 1e-5, 1e-5];  % fv fc D_Fn D_Qin D_Qon 1/beta\nTheta_Boom_Min = [10,  20, -200, 1/(1.25e9), -1e-5, -1e-5];\nTheta_Stick_Max = [100, 500, 200, 1/(2e8), 1e-5, 1e-5];  % fv fc D_Fn D_Qin D_Qon 1/beta\nTheta_Stick_Min = [10,  20, -200, 1/(1.25e9), -1e-5, -1e-5];\nTheta_Load_Max = 50;\nTheta_Load_Min = -Theta_Load_Max;\n\n% Apply parameter limits\nfor idx = 1:3\n    %Swing\n    Theta_Swing_F_hat_next(idx) = min(max(Theta_Swing_F_hat_next(idx), Theta_Swing_Min(idx)), Theta_Swing_Max(idx));\n    Theta_Swing_Q_hat_next(idx) = min(max(Theta_Swing_Q_hat_next(idx), Theta_Swing_Min(idx + 3)), Theta_Swing_Max(idx + 3));\n    \n    %Boom\n    Theta_Boom_F_hat_next(idx) = min(max(Theta_Boom_F_hat_next(idx), Theta_Boom_Min(idx)), Theta_Boom_Max(idx));\n    Theta_Boom_Q_hat_next(idx) = min(max(Theta_Boom_Q_hat_next(idx), Theta_Boom_Min(idx + 3)), Theta_Boom_Max(idx + 3));\n    \n    %Stick\n    Theta_Stick_F_hat_next(idx) = min(max(Theta_Stick_F_hat_next(idx), Theta_Stick_Min(idx)), Theta_Stick_Max(idx));\n    Theta_Stick_Q_hat_next(idx) = min(max(Theta_Stick_Q_hat_next(idx), Theta_Stick_Min(idx + 3)), Theta_Stick_Max(idx + 3));\n\n    %Load\n    Theta_Load_hat_next = min(max(Theta_Load_hat_next, Theta_Load_Min), Theta_Load_Max);\nend\n\n\nif  Use_Preset_Theta == 1\n    Theta_Swing_F_hat_next = [Theta_s1_init(1);Theta_s1_init(4);Theta_s1_init(7)];\n    Theta_Boom_F_hat_next = [Theta_s1_init(2);Theta_s1_init(5);Theta_s1_init(8)];\n    Theta_Stick_F_hat_next = [Theta_s1_init(3);Theta_s1_init(6);Theta_s1_init(9)];\n    Theta_Swing_Q_hat_next = [Theta_s2_init(1);Theta_s2_init(4);Theta_s2_init(7)];\n    Theta_Boom_Q_hat_next = [Theta_s2_init(2);Theta_s2_init(5);Theta_s2_init(8)];\n    Theta_Stick_Q_hat_next = [Theta_s2_init(3);Theta_s2_init(6);Theta_s2_init(9)];\n   % Theta_Load_hat_next    = 0;\nend\n\n\nif  Stop_Theta_Update == 1\n    Theta_Swing_F_hat_next = Theta_Swing_F_hat;\n    Theta_Boom_F_hat_next = Theta_Boom_F_hat;\n    Theta_Stick_F_hat_next = Theta_Stick_F_hat;\n    Theta_Swing_Q_hat_next = Theta_Swing_Q_hat;\n    Theta_Boom_Q_hat_next = Theta_Boom_Q_hat;\n    Theta_Stick_Q_hat_next = Theta_Stick_Q_hat;\n    Theta_Load_hat_next    = Theta_Load_hat;\nend\n%% ----------------------Gamma_Update----------------------\n% Update rates\nalpha_1 = 0.2;\nalpha_2 = 0.2;\nalpha_L = 0.2;\n\n% Calculate Gamma derivatives\nGamma_1_Swing_dot = alpha_1 * Gamma_1_Swing - xi_1(1) * Gamma_1_Swing * (F_Phi_Swing' * F_Phi_Swing) * Gamma_1_Swing;\nGamma_1_Boom_dot = alpha_1 * Gamma_1_Boom - xi_1(2) * Gamma_1_Boom * (F_Phi_Boom' * F_Phi_Boom) * Gamma_1_Boom;\nGamma_1_dot = alpha_1 * Gamma_1 - xi_1(3) * Gamma_1 * (F_Phi_Stick' * F_Phi_Stick) * Gamma_1;\n\nGamma_2_Swing_dot = alpha_2 * Gamma_2_Swing - xi_2(1) * Gamma_2_Swing * (Q_Phi_Swing' * Q_Phi_Swing) * Gamma_2_Swing;\nGamma_2_Boom_dot = alpha_2 * Gamma_2_Boom - xi_2(2) * Gamma_2_Boom * (Q_Phi_Boom' * Q_Phi_Boom)* Gamma_2_Boom;\nGamma_2_dot = alpha_2 * Gamma_2 - xi_2(3) * Gamma_2 * (Q_Phi_Stick' * Q_Phi_Stick) * Gamma_2;\n\nGamma_L_dot = alpha_L * Gamma_L - xi_L * Gamma_L * (phi_load_f' * phi_load_f) * Gamma_L;\n\n% Update Gamma matrices\nGamma_1_Swing_next = Gamma_1_Swing_dot * ts + Gamma_1_Swing;\nGamma_1_Boom_next = Gamma_1_Boom_dot * ts + Gamma_1_Boom;\nGamma_1_next = Gamma_1_dot * ts + Gamma_1;\n\nGamma_2_Swing_next = Gamma_2_Swing_dot * ts + Gamma_2_Swing;\nGamma_2_Boom_next = Gamma_2_Boom_dot * ts + Gamma_2_Boom;\nGamma_2_next = Gamma_2_dot * ts + Gamma_2;\n\nGamma_L_next = Gamma_L_dot * ts + Gamma_L;\n\n% Gamma limits\nGamma_1_Max = [1000, 1000, 1000];\nGamma_1_Min = -Gamma_1_Max;\nGamma_2_Max = [1e-1, 1e-3, 1e-3];\nGamma_2_Min = -Gamma_2_Max;\nGamma_L_Max = 5;\nGamma_L_Min = -Gamma_L_Max;\n\n% Apply Gamma limits\nfor idx = 1:3\n    % Swing\n    Gamma_1_Swing_next  = min(max(Gamma_1_Swing_next , Gamma_1_Min(idx)), Gamma_1_Max(idx));\n    Gamma_2_Swing_next  = min(max(Gamma_2_Swing_next , Gamma_2_Min(idx)), Gamma_2_Max(idx));\n    \n    % Boom\n    Gamma_1_Boom_next  = min(max(Gamma_1_Boom_next , Gamma_1_Min(idx)), Gamma_1_Max(idx));\n    Gamma_2_Boom_next  = min(max(Gamma_2_Boom_next , Gamma_2_Min(idx)), Gamma_2_Max(idx));\n    \n    % Stick\n    Gamma_1_next = min(max(Gamma_1_next , Gamma_1_Min(idx)), Gamma_1_Max(idx));\n    Gamma_2_next  = min(max(Gamma_2_next , Gamma_2_Min(idx)), Gamma_2_Max(idx));\n\n    Gamma_L_next = min(max(Gamma_L_next , Gamma_L_Min), Gamma_L_Max);\nend\n\n\n%% ----------------------dihat_Updata----------------------\n\nd1hat_dot = diag(gamma_d1) * e2;\nd2hat_dot = diag(gamma_d2) * e3;\nd1hat_next = d1hat_dot * ts + d1hat(:);\nd2hat_next = d2hat_dot * ts + d2hat(:);\nd1max = ones(3 ,1) * 1e2;\nd2max = ones(3 ,1) * 5e-4;\nd1min = -d1max;\nd2min = -d2max;\nfor idx = 1 : 3\n   if d1hat_next(idx) > d1max(idx)\n       d1hat_next(idx) = d1max(idx);\n   end\n    if d1hat_next(idx) < d1min(idx)\n       d1hat_next(idx) = d1min(idx);\n   end\n\n   if d2hat_next(idx) > d2max(idx)\n       d2hat_next(idx) = d2max(idx);\n    end\n    if d2hat_next(idx) < d2min(idx)\n       d2hat_next(idx) = d2min(idx);\n    end\nend\nif sw_d1hat == 0\n    d1hat_next = zeros(3,1);\n    d1hat_dot  = 0;\nend\nif sw_d2hat == 0\n    d2hat_next = zeros(3,1);\n    d2hat_dot  = 0;\nend\n\n%%\n% Q to U\nPr = 0;                                     \nkq1 = 1.069e-9;                         \t\nkq2 = 1.069e-9;                           \t\nk = 10;                                    \t\n\nif QLd > 0 % forword\n    Delta_p1 = Ps - Pi;\n    Delta_p2 = Po - Pr;\nelse % backspacings\n    Delta_p1 = Pi - Pr;\n    Delta_p2 = Ps - Po;\nend\n\nXv = QLd ./ (Ai./Vi.*kq1.*sqrt(Delta_p1) + Ao./Vo.*kq2.*sqrt(Delta_p2));\nU = 1./k .* Xv;          \n\nUmax = 5;\nfor idx = 1 : 3\n    if U(idx) > Umax\n        U(idx) = Umax;\n    end\n    if U(idx) < -Umax\n        U(idx) = -Umax;\n    end\nend\n\n\n\n\n%%  ————————detect——————————\nF_Swing = [FLd(1); FLda1(1); FLds1(1); FLda2(1)];\nF_Boom  = [FLd(2); FLda1(2); FLds1(2); FLda2(2)];\nF_Stick = [FLd(3); FLda1(3); FLds1(3); FLda2(3)];\n\n% Q组\nQ_Swing = [QLd(1); QLda1(1); QLds1(1); QLda2(1)];\nQ_Boom  = [QLd(2); QLda1(2); QLds1(2); QLda2(2)];\nQ_Stick = [QLd(3); QLda1(3); QLds1(3); QLda2(3)];\n\ntau = J_h * FL;" ("Base Controller")("q1"=w363, "q2"=w325, "q3"=w324, "alpha1"=w361, "alpha2"=w360, "alpha3"=w357, "pi1"=w355, "pi2"=w346, "pi3"=w347, "po1"=w348, "po2"=w349, "po3"=w350, "ts"=w337, "Ps"=w345, "Desired_Swing"=w328, "Desired_Boom"=w327, "Desired_Stick"=w326, "K1"="K1", "K2"="K2", "K3"=w313, "q_dot_f"=w267, "q_f"=w268, "Desired_q_Swing"=w321, "Desired_q_Boom"=w322, "Desired_q_Stick"=w323, "sw_QLda1"="sw_QLda1", "sw_FLda1"="sw_FLda1", "Theta_s1_init"="Theta_s1_init", "Theta_s2_init"=w306, "gamma_d1"="gamma_d1", "gamma_d2"=w316, "d1hat"=w312, "d2hat"=w310, "sw_d1hat"="sw_d1hat", "sw_d2hat"="sw_d2hat", "X1_f"=w305, "X2_f"=w304, "Gamma_1"=w255, "Theta_Stick_F_hat"=w299, "Gamma_2"=w253, "Theta_Stick_Q_hat"=w297, "Gamma_1_Swing"=w263, "Gamma_1_Boom"=w259, "Gamma_2_Swing"=w261, "Gamma_2_Boom"=w257, "Theta_Swing_F_hat"=w295, "Theta_Swing_Q_hat"=w293, "Theta_Boom_Q_hat"=w290, "Theta_Boom_F_hat"=w291, "w1"="w1", "w2"="w2", "sw_Y_Q"="sw_Y_Q", "Stop_Theta_Update"="Stop\nTheta_Update", "Use_Preset_Theta"="Use\nPreset_Theta", "Gamma_L"=w219, "Theta_Load_hat"=w217) -> ("q_dot_f_next"=w264:dbl[], "q_f_next"=w265:dbl[], "U"=w333:dbl[], "d1hat_next"=w311:dbl[], "d2hat_next"=w309:dbl[], "X2_f_next"=w303:dbl[], "X1_f_next"=w302:dbl[], "Gamma_1_next"=w254:dbl, "Theta_Stick_F_hat_next"=w243:dbl[], "Theta_Stick_Q_hat_next"=w240:dbl[], "Gamma_2_next"=w252:dbl, "Gamma_1_Swing_next"=w262:dbl, "Gamma_2_Swing_next"=w260:dbl, "Gamma_1_Boom_next"=w258:dbl, "Gamma_2_Boom_next"=w256:dbl, "Theta_Swing_F_hat_next"=w294:dbl[], "Theta_Swing_Q_hat_next"=w292:dbl[], "Theta_Boom_Q_hat_next"=w236:dbl[], "Theta_Boom_F_hat_next"=w237:dbl[], "Epsilon_1"=w286:cdb[], "Epsilon_2"=w284:cdb[], "e2"=→"e2":dbl[], "e3"=→"e3":dbl[], "tau"=w222:dbl[], "F_Swing"=w283:cdb[], "F_Boom"=w274:cdb[], "F_Stick"=w273:cdb[], "Q_Swing"=w275:cdb[], "Q_Stick"=w277:cdb[], "Q_Boom"=w276:cdb[], "e2_e3"=→"e2_e3":dbl[], "Gamma_L_next"=w214:cdb, "Theta_Load_hat_next"=w215:cdb)  [unwired: 1 in, 1 out]
    "ARC_U" <- w333
    "Theta_Stick_F_hat_next" <- w243
    "Theta_Stick_Q_hat_next" <- w240
    "Theta_Swing_F_hat_next" <- w294
    "Theta_Swing_Q_hat_next" <- w292
    "Theta_Boom_F_hat_next" <- w237
    "Theta_Boom_Q_hat_next" <- w236
    "Load" <- w215
    "Gamma_L" <- w214
    n192 = shared-variable ".\\sharedV.lvlib\\Actual_tau"(w222) -> ()  [unwired: 1 in, 1 out]
    n193 = Array To Cluster ("数组至簇转换")(array=w277) -> (cluster=→"Q_Stick":T11)
    n194 = Array To Cluster ("数组至簇转换")(array=w276) -> (cluster=→"Q_Boom":T12)
    n195 = Array To Cluster ("数组至簇转换")(array=w275) -> (cluster=→"Q_Swing":T13)
    n196 = Array To Cluster ("数组至簇转换")(array=w273) -> (cluster=→"F_Stick":T14)
    n197 = Array To Cluster ("数组至簇转换")(array=w274) -> (cluster=→"F_Boom":T15)
    n198 = Array To Cluster ("数组至簇转换")(array=w283) -> (cluster=→"F_Swing":T16)
    n199 = feedback-in #4(w265) -> ()
    n200 = feedback-in #5(w264) -> ()
    n201 = feedback-in #6(w237) -> ()
    n202 = feedback-in #7(w236) -> ()
    n203 = feedback-in #8(w292) -> ()
    n204 = feedback-in #9(w240) -> ()
    n205 = feedback-in #10(w214) -> ()
    n206 = feedback-in #11(w262) -> ()
    n207 = feedback-in #12(w260) -> ()
    n208 = feedback-in #13(w258) -> ()
    n209 = feedback-in #14(w256) -> ()
    n210 = feedback-in #15(w254) -> ()
    n211 = feedback-in #16(w252) -> ()
    n212 = feedback-in #17(w294) -> ()
    n213 = feedback-in #18(w243) -> ()
    n214 = feedback-in #19(w215) -> ()
    n215 = feedback-in #20(w311) -> ()
    n216 = feedback-in #21(w309) -> ()
    n217 = feedback-in #22(w302) -> ()
    n218 = feedback-in #23(w303) -> ()
    n219 = Array Size ("数组大小")(array=w333) -> ()  [unwired: 1 out]
    n220 = Index Array ("索引数组")(array=w333, index=1) -> (element=w329:dbl)
    n221 = Index Array ("索引数组")(array=w333, index=0) -> (element=w334:dbl)
    n222 = Index Array ("索引数组")(array=w333, index=2) -> (element=w330:dbl)
    n223 = shared-variable ".\\sharedV.lvlib\\ARC_U_Swing"(w334) -> ()  [unwired: 1 in, 1 out]
    n224 = Array To Cluster ("数组至簇转换")(array=w286) -> (cluster=→"Esti_e1":T17)
    n225 = Array To Cluster ("数组至簇转换")(array=w284) -> (cluster=→"Esti_e2":T18)
    n226 = expression code="(x/pi)*180.0" ("弧度转换至角度")(w265) -> (w220:dbl[])
    n227 = expression code="(x/pi)*180.0" ("弧度转换至角度")(w264) -> (w221:dbl[])
    n228 = shared-variable ".\\sharedV.lvlib\\load"(w215) -> ()  [unwired: 1 in, 1 out]
    n229 = shared-variable ".\\sharedV.lvlib\\ARC_U_Boom"(w329) -> ()  [unwired: 1 in, 1 out]
    n230 = shared-variable ".\\sharedV.lvlib\\ARC_U_Stick"(w330) -> ()  [unwired: 1 in, 1 out]
    n231 = shared-variable ".\\sharedV.lvlib\\q_dot_f"(w221) -> ()  [unwired: 1 in, 1 out]
    n232 = shared-variable ".\\sharedV.lvlib\\q_f"(w220) -> ()  [unwired: 1 in, 1 out]
    n233 = Array To Cluster ("数组至簇转换")(array=w240) -> (cluster=→"Theta_Stick_Q_hat_next":T19)
    n234 = Array To Cluster ("数组至簇转换")(array=w243) -> (cluster=→"Theta_Stick_F_hat_next":T1)
    n235 = Array To Cluster ("数组至簇转换")(array=w236) -> (cluster=→"Theta_Boom_Q_hat_next":T20)
    n236 = Array To Cluster ("数组至簇转换")(array=w237) -> (cluster=→"Theta_Boom_F_hat_next":T21)
    n237 = node-c288() -> ()  [unwired: 1 in, 1 out]
  }
  n238 = node-c288(w8) -> ()  [unwired: 1 out]
